vi "BLE v2.0-scalable.vi"(7 "Est Thresh Val":dbl, 8 "Threshold Value Analysis":bool, 9 "Model Name":string="model_name", 10 "Ex_Mod_IDs":string[](array[string]), 11 "Sp_Id_Arr":string[](array[string])) -> (0 "Close 2":bool, 3 "Boolean  Expression":string)   [LabVIEW 2014]
uses:
  <vilib>/Utility/file.llb/Read From Spreadsheet File (string).vi
  <vilib>/Utility/file.llb/Read From Spreadsheet File (DBL).vi
  <vilib>/regexp/Match Regular Expression.xnode
panel:
  out "Input File":path=path "/Volumes/Macintosh HD/Users/hasan/My_MAC_Data/3_Dissemination/DATE 2017/Experimentation/Experimental Results/6Gx78/x78_SSADataLog.xls"
  out "Estimation Time (s)":dbl
  out "Compare":i32[](array[numeric])
  out "element":bool
  out "Output Array":bool[](array[boolean])
  out "Final_BE":string
  out "Int_BE":string
  out "Array 2":bool[][](array[boolean])
  out "Dig_In":bool[](array[boolean])
  out "TV":dbl
  out "Array":u32[](array[numeric])
  out "output variable":i32[](array[numeric])
  out "SD":i32
  out "OP_Var":i32[](array[numeric])
  out "HIGH":i32[](array[numeric])
  out "icv":i32
  out "Case_O":i32[][](array[numeric])
  out "Case_I":i32[](array[numeric])
  out "nc":i32
  out "Input Status":bool
  out "% fitness":string
  out "Simulation Data":string[][](table)
  in  "Close":bool
  out "Row header":string[](array[string])
  out "N":i32
  out "Thresh Val":dbl[](array[numeric])
  out "All Data":string[][](array[string])
  out "Analog Data":dbl[][](array[numeric])
  out "All Data":dbl[][](array[numeric])
  out "Index":i32[](array[numeric])
  out "C1_Ar":dbl[](array[numeric])
  out "C2_Ar":dbl[](array[numeric])
  out "C3_Ar":dbl[](array[numeric])
  out "C4_Ar":dbl[](array[numeric])
  out "Cs4_1s":i32
  out "Cs3_1s":i32
  out "Cs2_1s":i32
  out "Cs1_1s":i32
  out "var_4":i8
  out "var_3":i8
  out "var_2":i8
  out "var_1":i8
  out "case4":i32
  out "case3":i32
  out "case2":i32
  out "case1":i32
  out "C4":dbl
  out "C3":dbl
  out "C2":dbl
  out "C1":dbl
  out "Digital Data":bool[][](array[boolean])
  # "Logic Expression"
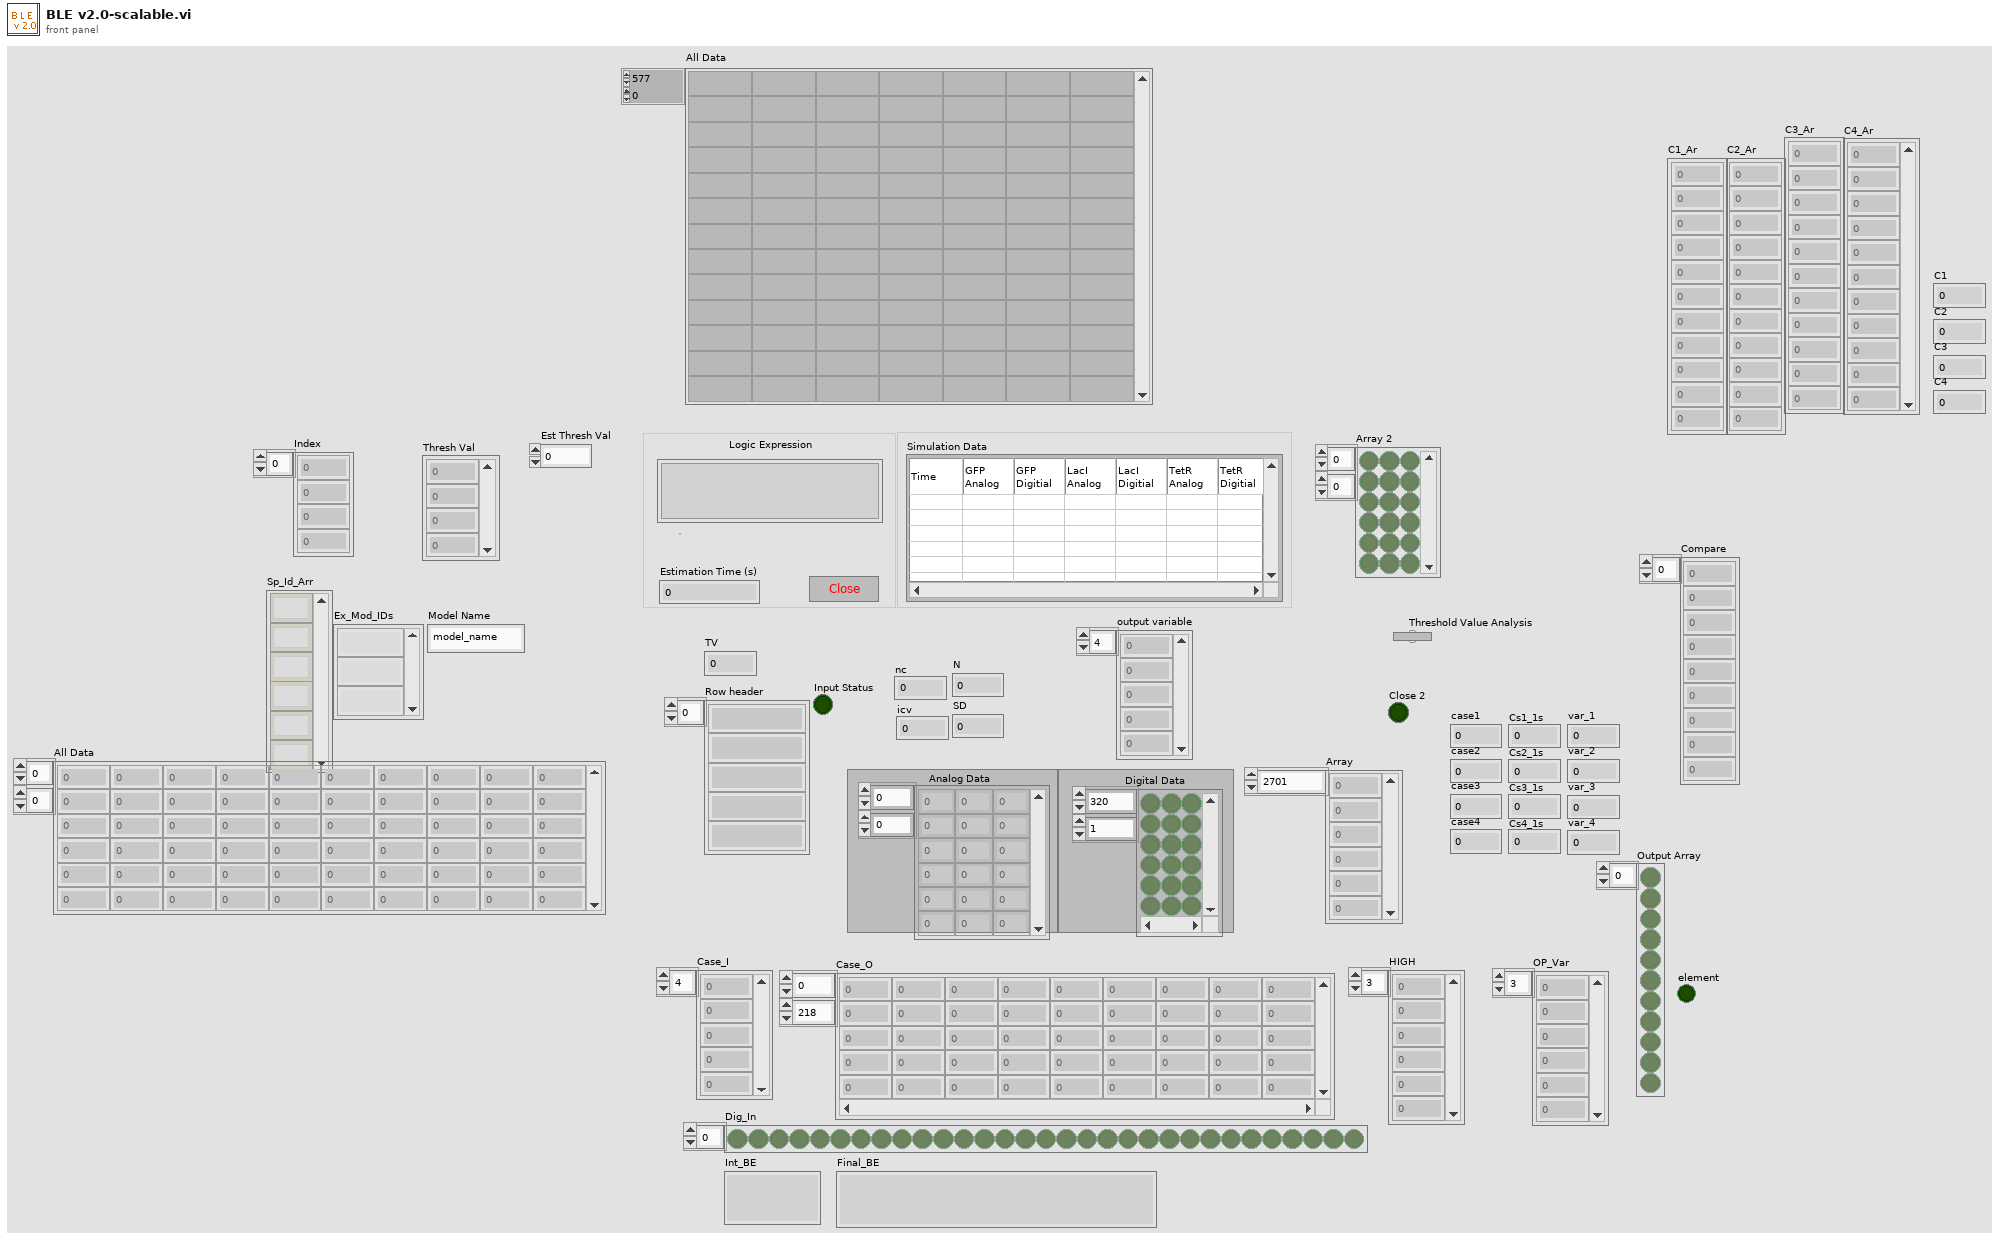
[diagram p1: front panel]
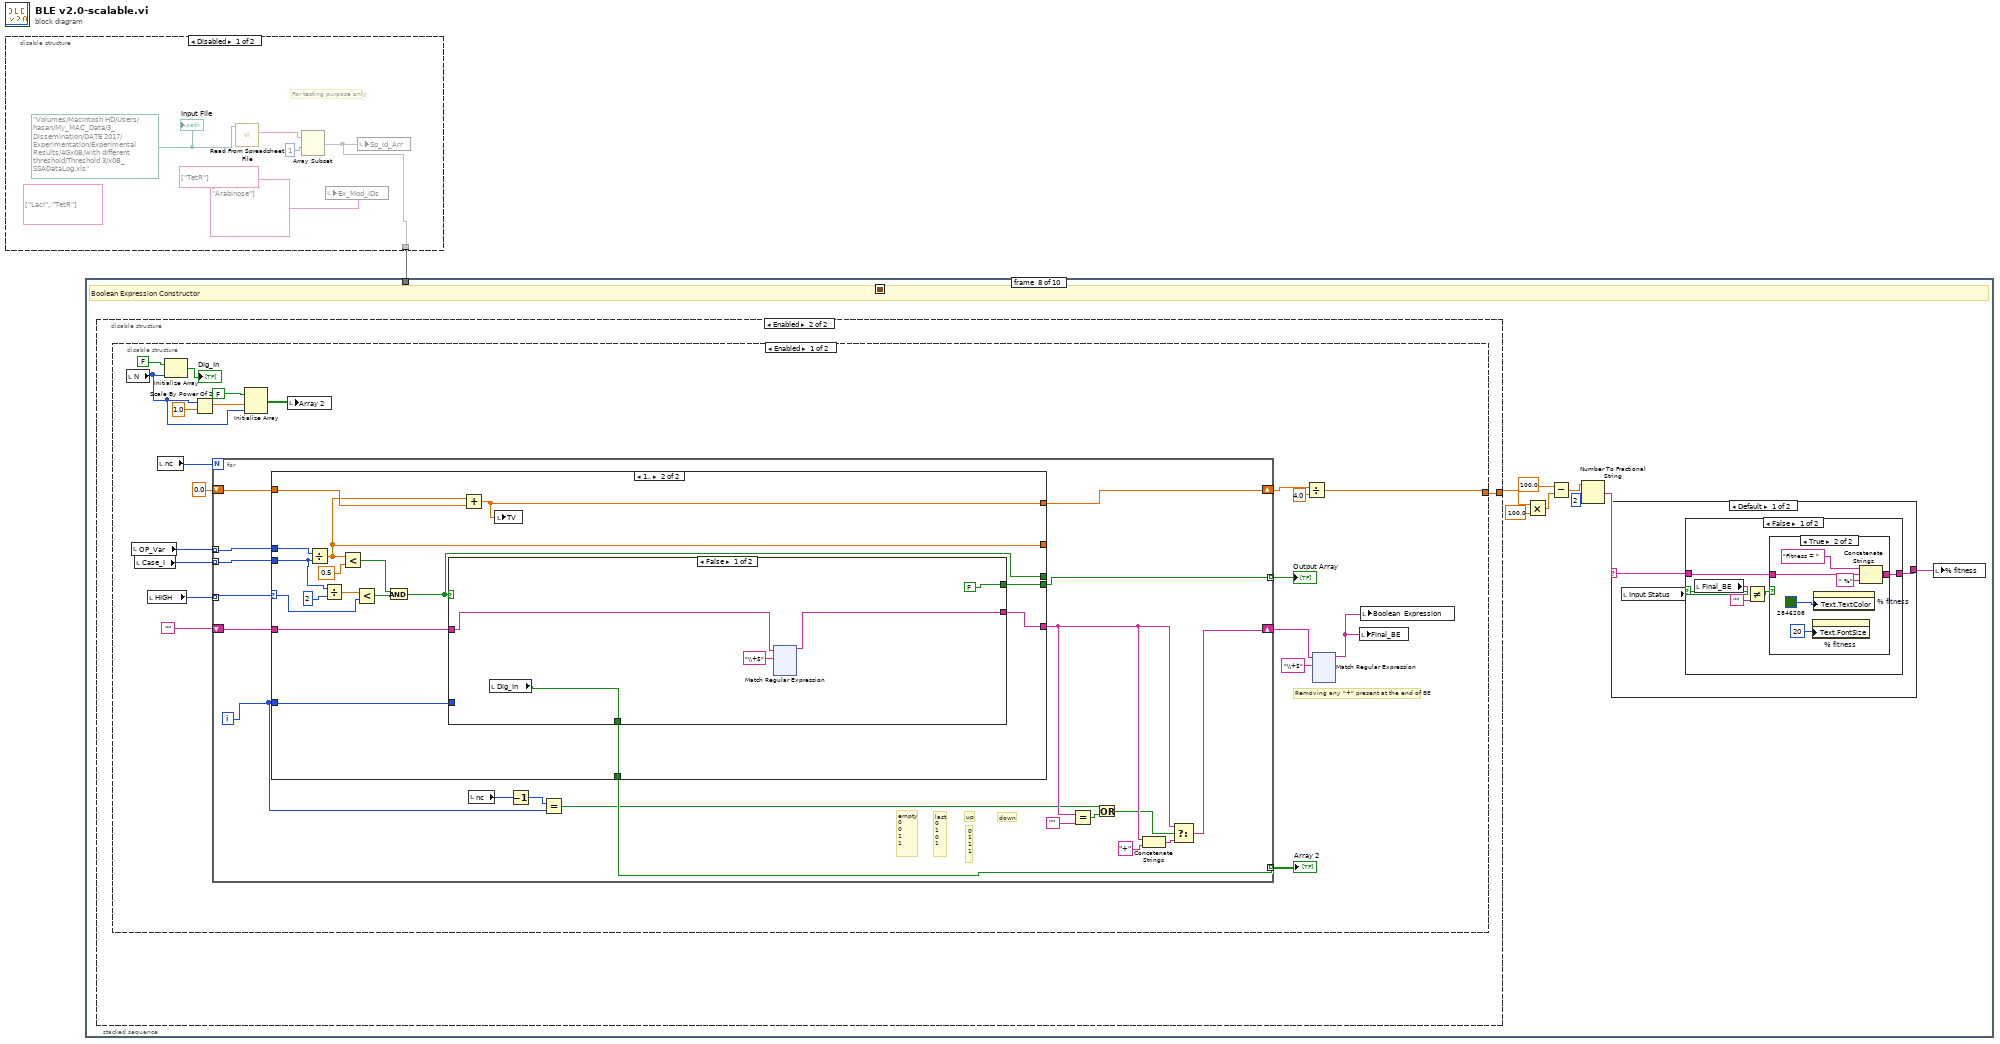
[diagram p0: block diagram]
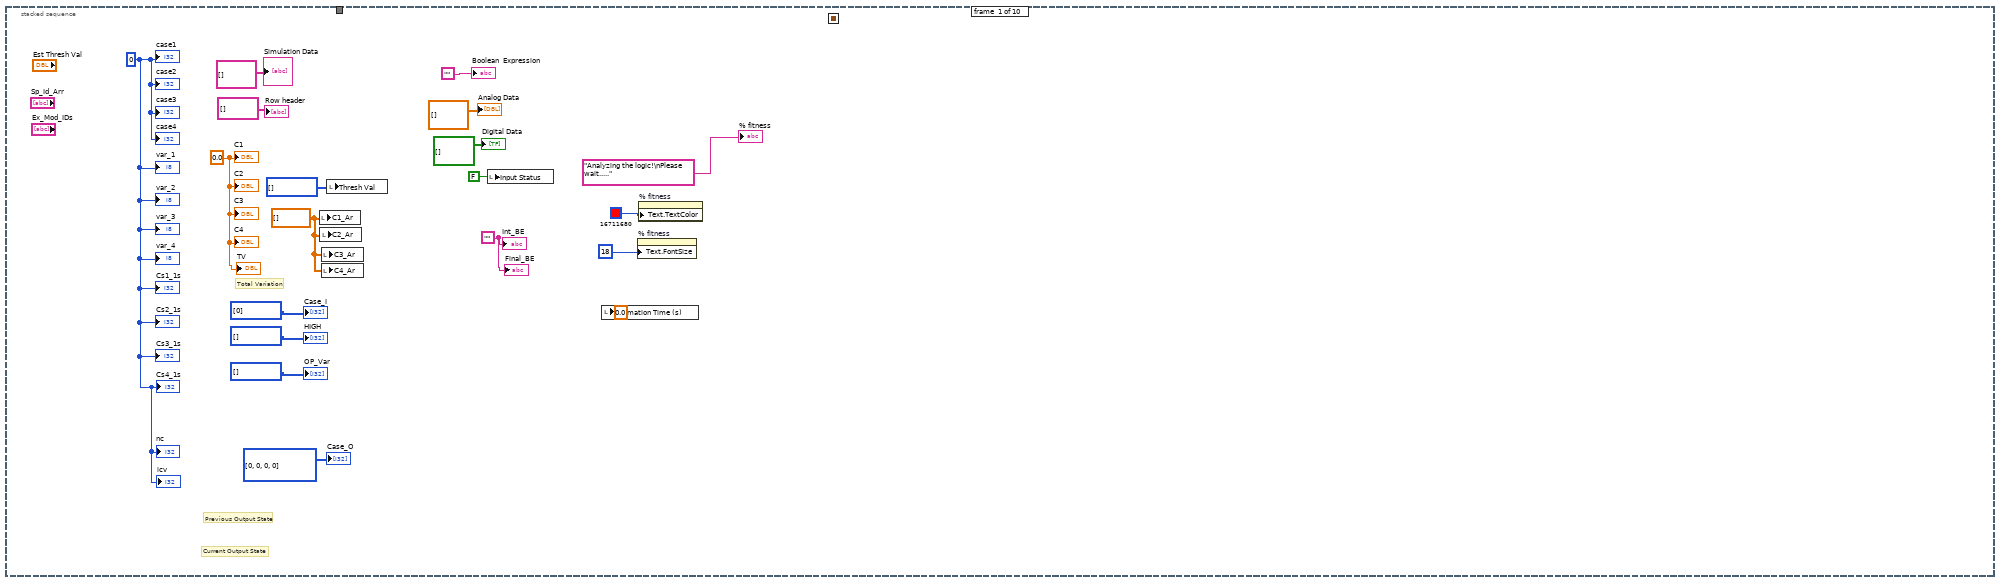
[diagram p3: hidden frame]
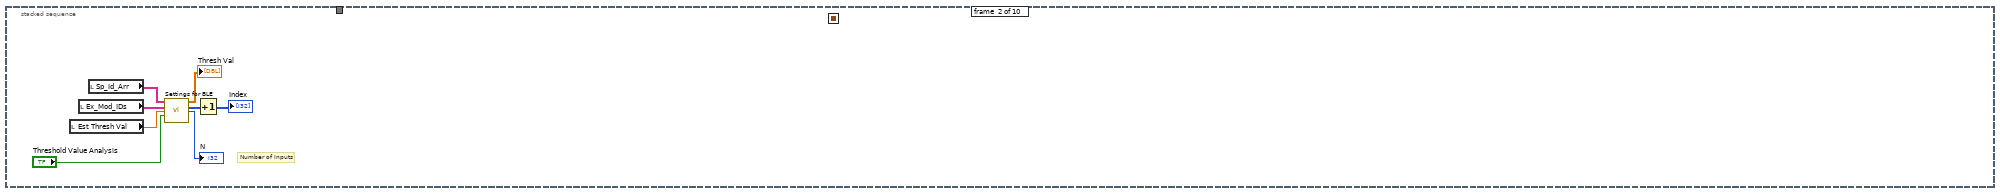
[diagram p4: hidden frame]
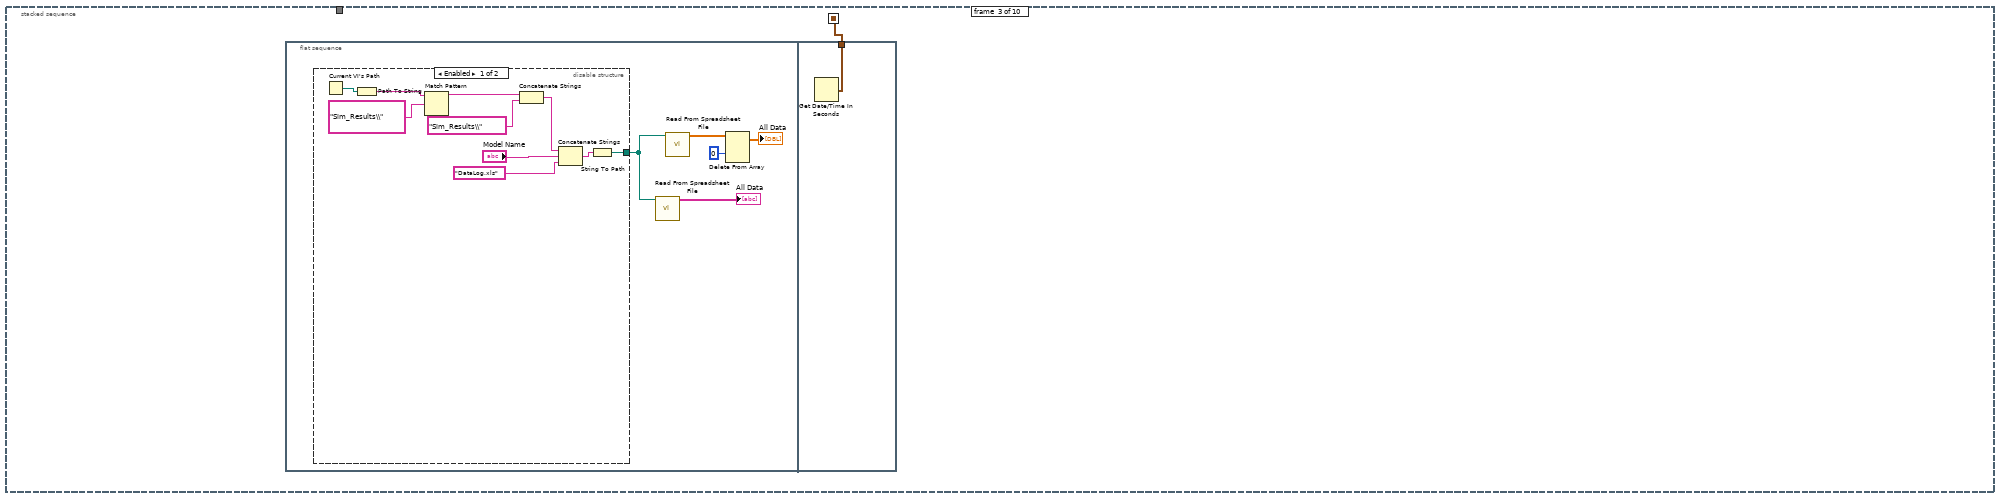
[diagram p5: hidden frame]
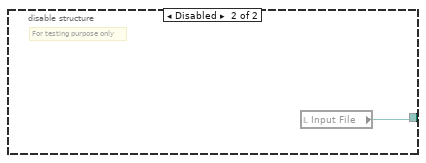
[diagram p6: hidden frame]
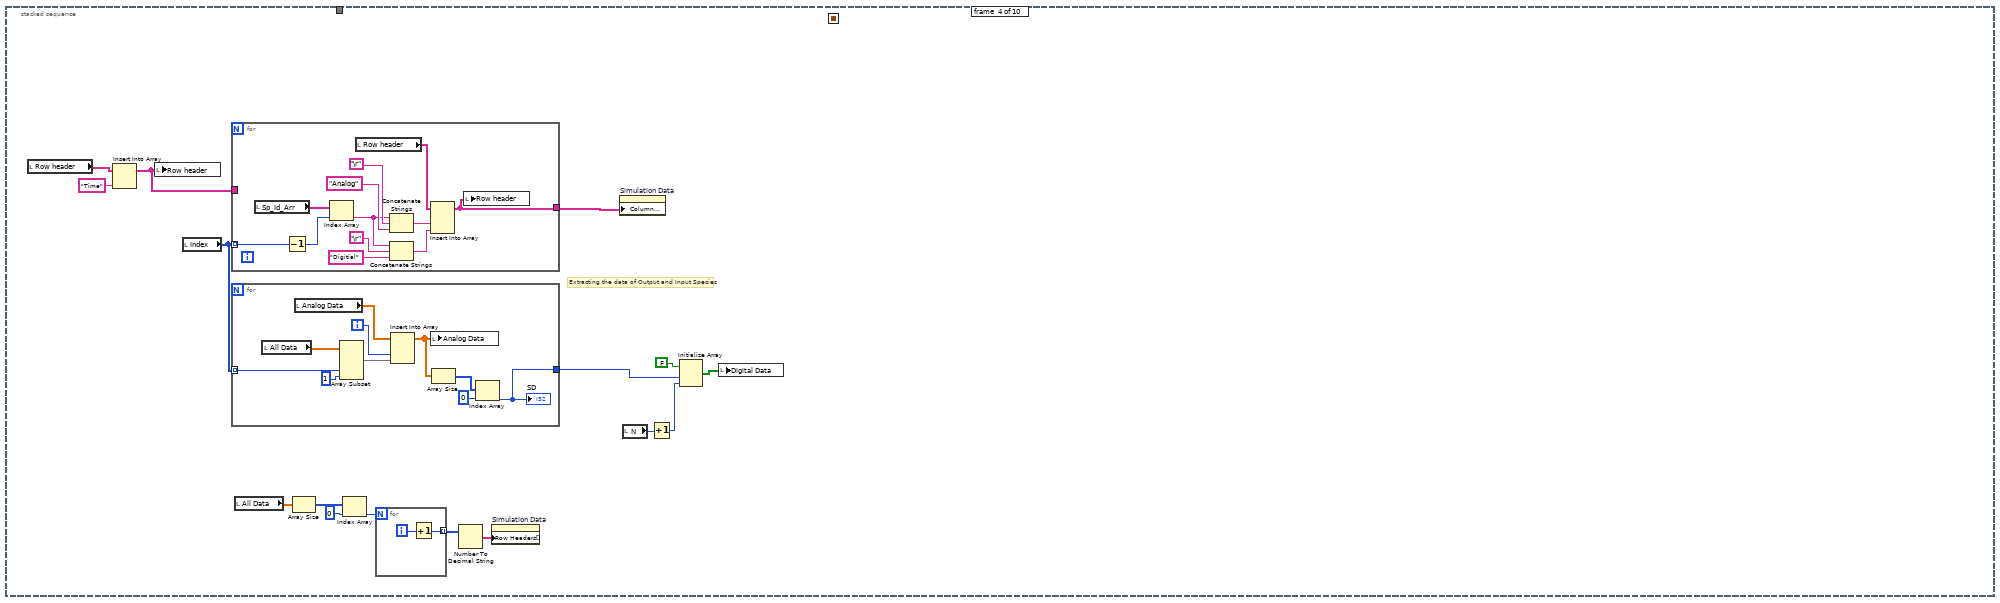
[diagram p7: hidden frame]
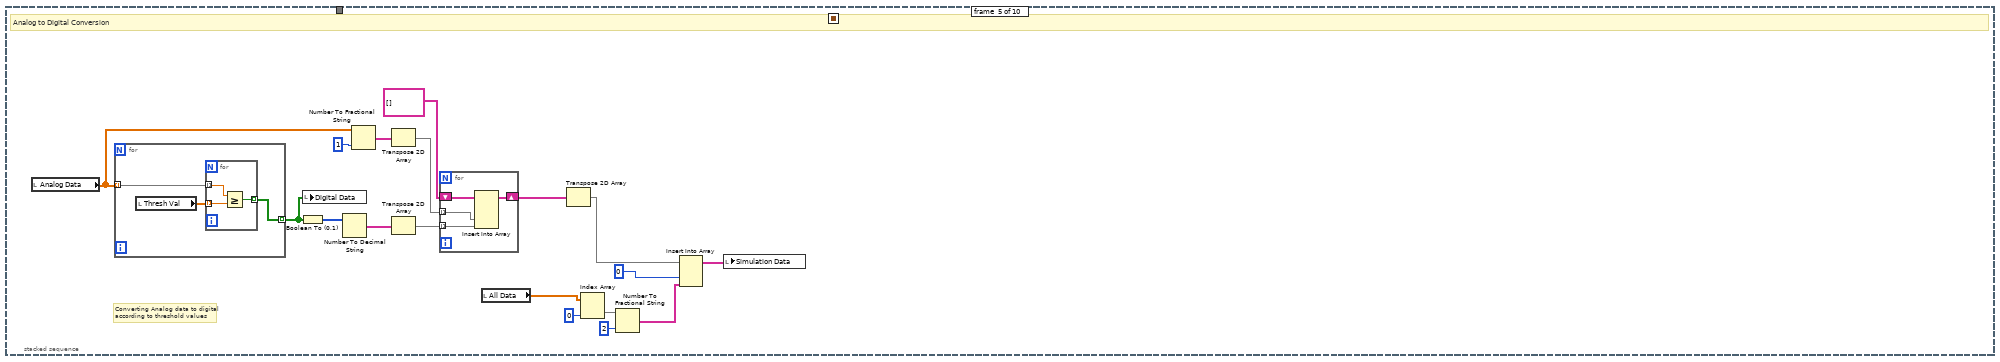
[diagram p8: hidden frame]
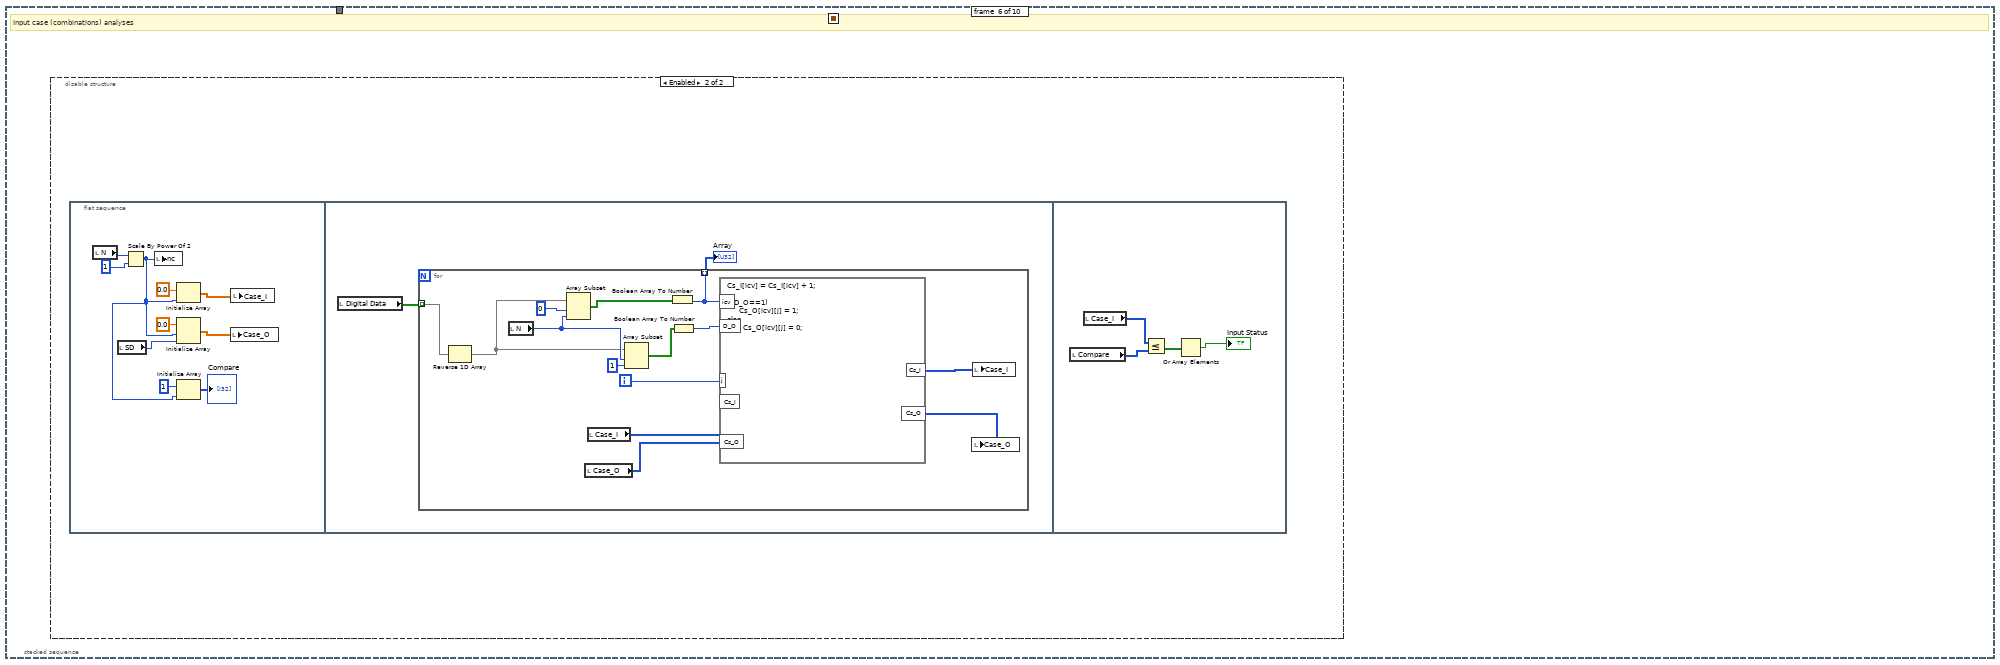
[diagram p9: hidden frame]
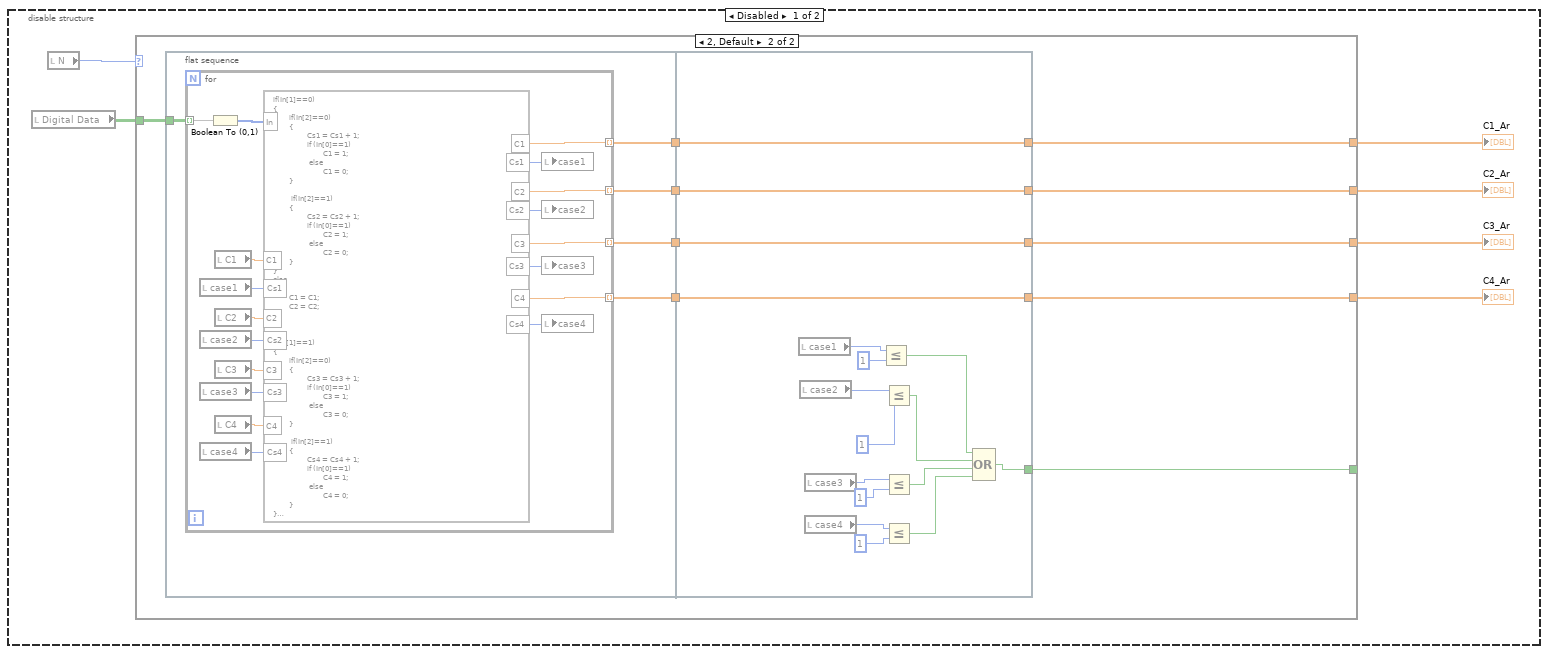
[diagram p10: hidden frame]
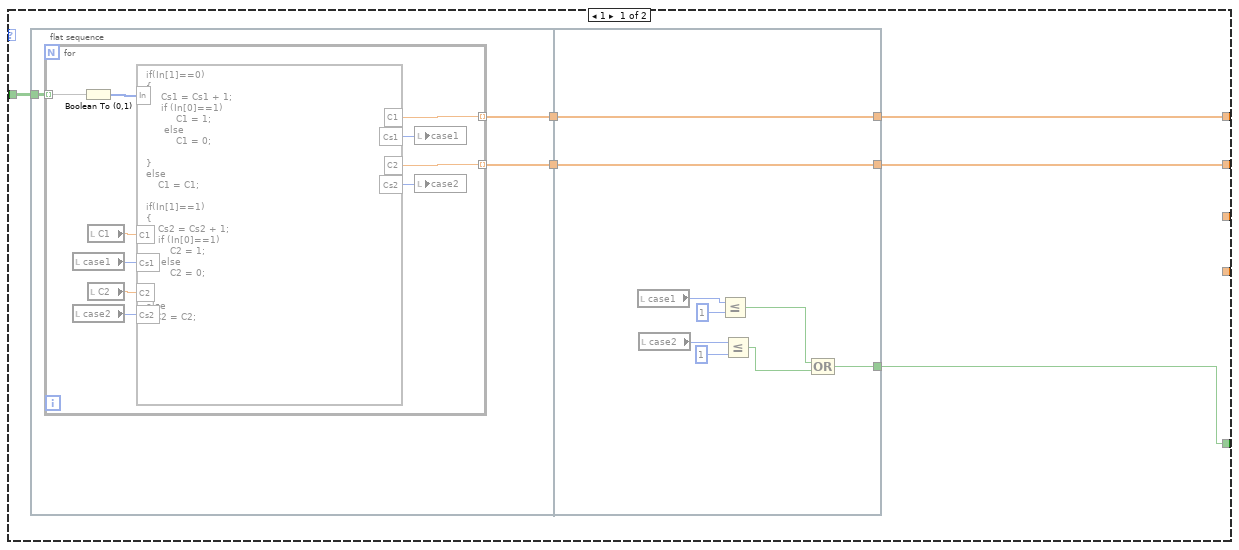
[diagram p11: hidden frame]
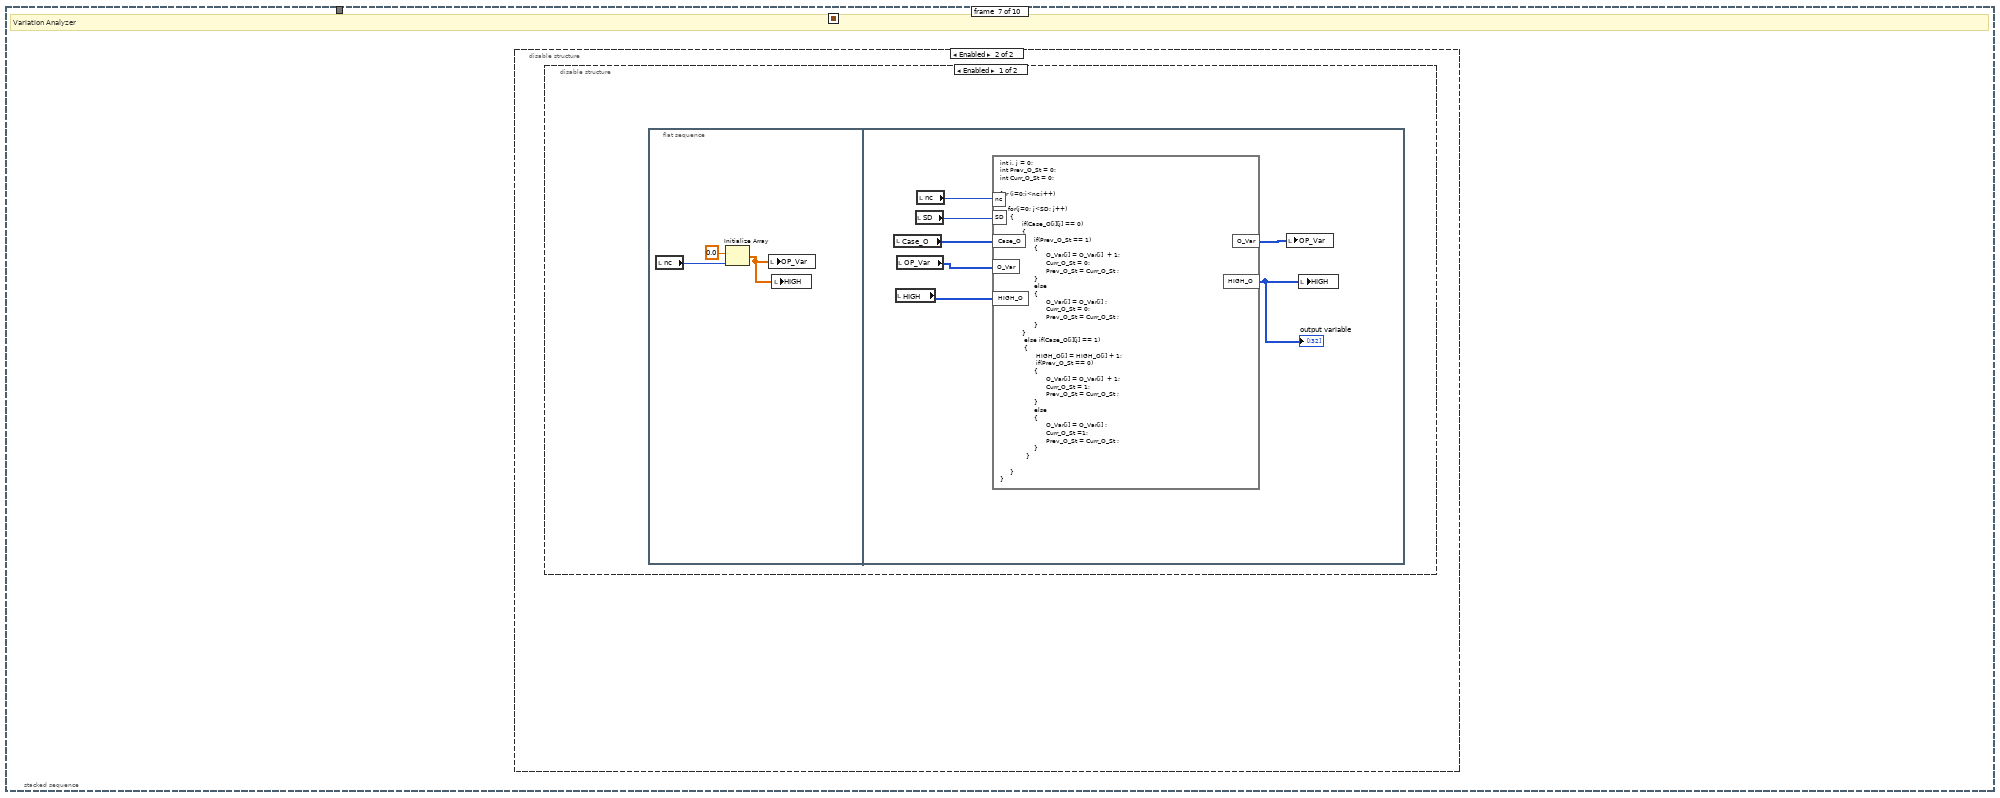
[diagram p12: hidden frame]
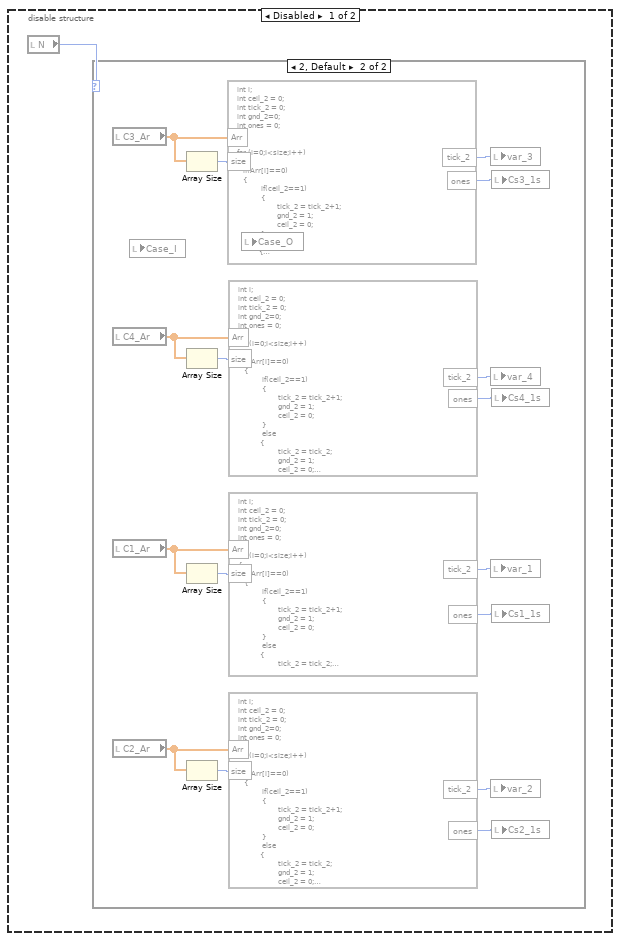
[diagram p13: hidden frame]
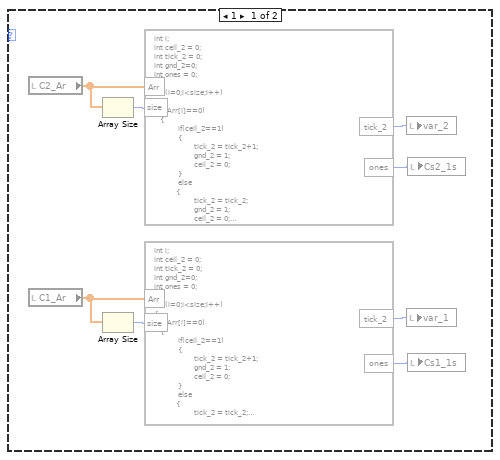
[diagram p14: hidden frame]
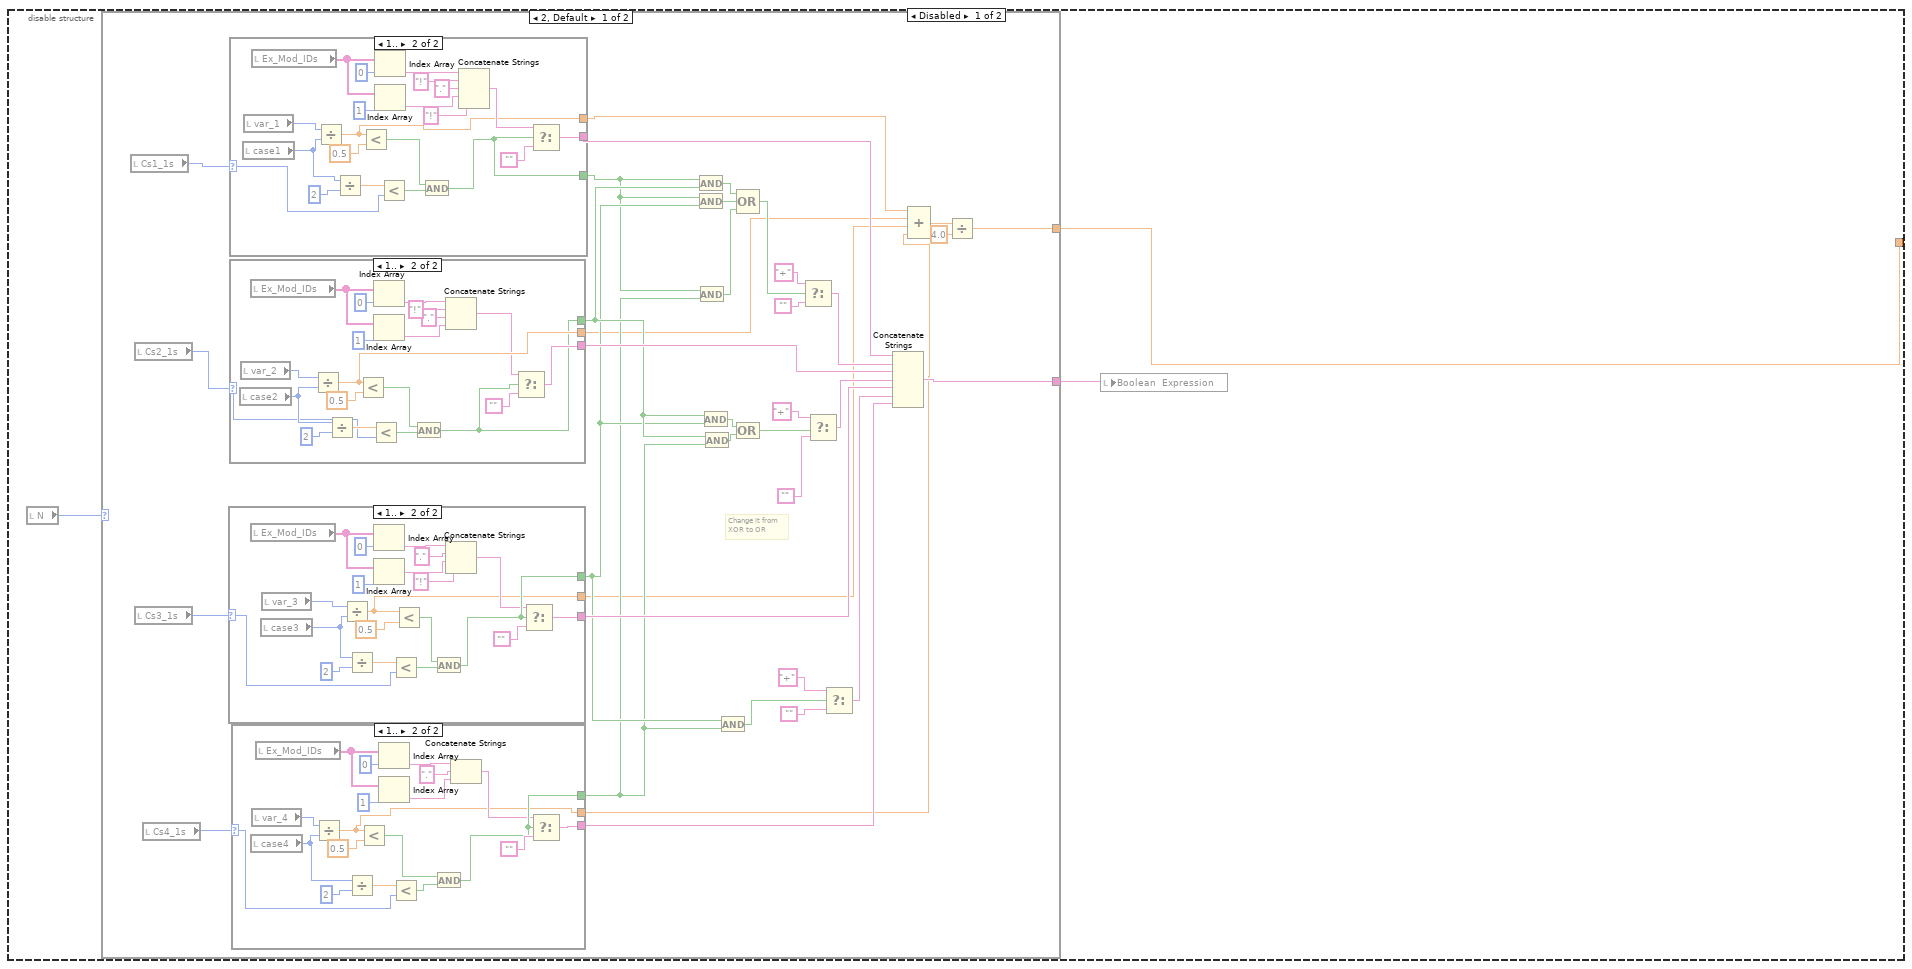
[diagram p16: hidden frame]
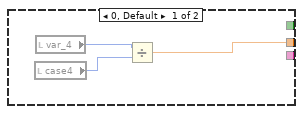
[diagram p17: hidden frame]
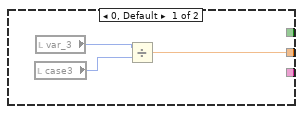
[diagram p18: hidden frame]
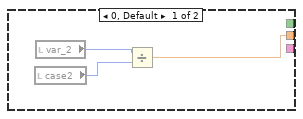
[diagram p19: hidden frame]
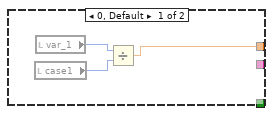
[diagram p20: hidden frame]
diagram:
  n1 = disable-structure shown="Disabled" {
    disable-tunnel: [w3 _] -> w1
    frame Disabled {
      (unwired) string[] ["LacI", "TetR"] ("Ex_Mod_IDs")
      (unwired) string[] ["TetR"] ("Ex_Mod_IDs")
      w6 = path "/Volumes/Macintosh HD/Users/hasan/My_MAC_Data/3_Dissemination/DATE 2017/Experimentation/Experimental Results/4Gx0B/with different threshold/Threshold 3/x0B_SSADataLog.xls"
      # "For testing purpose only"
      n2 = call-poly <vilib>:"Read From Spreadsheet File.vi"("file path (dialog if empty)"=w6) -> ("first row"=w5:string[])  [unwired: 6 in, 4 out]
      n3 = Array Subset(array=w5, index=1) -> (w3:string[])  [unwired: 1 in]
      n4 = local write "Ex_Mod_IDs"(string[] ["IPTG", "aTc", "Arabinose"] ("Ex_Mod_IDs")) -> ()
      n5 = local write "Sp_Id_Arr"(w3) -> ()
      "Input File" <- w6
    }
    frame Enabled {
    }
  }
  n6 = stacked-sequence {
    seq-local: [_ _ w34 _ _ _ _ _ _ _] -> [_ _ _ _ _ _ _ _ _ w1069]
    tunnel: w1 -> [_ _ _ _ _ _ _ _ _ _]
    frame #0 {
      w11 = ""
      w12 = 0.0 ("C1")
      w13 = 0 ("case1")
      w22 = dbl[] [] ("C1_Ar")
      # "Total Variation"
      # "Current Output State"
      # "Previous Output State"
      n7 = local write "C1_Ar"(w22) -> ()
      n8 = local write "C2_Ar"(w22) -> ()
      n9 = local write "C3_Ar"(w22) -> ()
      n10 = local write "C4_Ar"(w22) -> ()
      n11 = local write "Thresh Val"(i32[] [] ("Array")) -> ()
      n12 = local write "Input Status"(FALSE ("Input Status")) -> ()
      n13 = local write "Estimation Time (s)"(0.0 ("x-y")) -> ()
      n14 = property on="% fitness" class="Str"("Text.FontSize"=u32 18 ("Text.Font:Size")) -> ()  [unwired: 2 in, 2 out]
      n15 = property on="% fitness" class="Str"("Text.TextColor"=u32 16711680) -> ()  [unwired: 2 in, 2 out]
      "C1" <- w12
      "C2" <- w12
      "C3" <- w12
      "C4" <- w12
      "case1" <- w13
      "case2" <- w13
      "case3" <- w13
      "case4" <- w13
      "var_1" <- w13
      "var_2" <- w13
      "var_3" <- w13
      "var_4" <- w13
      "Cs1_1s" <- w13
      "Cs2_1s" <- w13
      "Cs3_1s" <- w13
      "Cs4_1s" <- w13
      "Simulation Data" <- string[][] [] ("Table Control")
      "Row header" <- string[] [] ("Row header 2")
      "Digital Data" <- bool[][] [] ("Dig. Data to Process")
      "Boolean  Expression" <- ""
      "Analog Data" <- dbl[][] [] ("Data to process")
      "% fitness" <- "Analyzing the logic!\nPlease wait....." ("% fitness")
      "nc" <- w13
      "Case_I" <- i32[] [0] ("Array")
      "Case_O" <- i32[][] [[0, 0], [0, 0]] ("Array")
      "icv" <- w13
      "HIGH" <- i32[] [] ("Array")
      "OP_Var" <- i32[] [] ("Array")
      "TV" <- w12
      "Int_BE" <- w11
      "Final_BE" <- w11
    }
    frame #1 {
      # "Number of Inputs"
      n16 = local read "Est Thresh Val"() -> (w27:dbl)
      n17 = local read "Ex_Mod_IDs"() -> (w32:string[])
      n18 = local read "Sp_Id_Arr"() -> (w33:string[])
      n19 = call "Settings for BLE.vi"("Sp_Id_Arr"=w33, "Ex_Mod_IDs"=w32, "Est Thresh Val"=w27, "Threshold Value Analysis"="Threshold Value Analysis") -> ("Thresh Val"=→"Thresh Val":dbl[], "Index"=w31:i32[], "No of I/ps"=→"N":i32)  [unwired: 9 in]
      n20 = Increment(x=w31) -> (x+1=→"Index":i32[])
    }
    frame #2 {
      n21 = flat-sequence {
        tunnel: [w51] -> w34
        frame #0 {
          n22 = disable-structure shown="Enabled" {
            disable-tunnel: [w49 w50] -> w39
            frame Enabled {
              n23 = Current VI's Path() -> (path=w46:path)
              n24 = Path To String(path=w46) -> (string=w45:string)
              n25 = Match Pattern(string=w45, regular expression="Sim_Results\\" ("string")) -> (before substring=w43:string)  [unwired: 1 in, 3 out]
              n26 = Concatenate Strings(w43, "Sim_Results\\" ("string")) -> (w47:string)
              n27 = Concatenate Strings(w47, "Model Name", "DataLog.xls" ("name or relative path")) -> (w48:string)
              n28 = String To Path(string=w48) -> (path=w49:path)
            }
            frame Disabled {
              # "For testing purpose only"
              n29 = local read "Input File"() -> (w50:path)
            }
          }
          n30 = call-poly <vilib>:"Read From Spreadsheet File.vi"("file path (dialog if empty)"=w39) -> ("all rows"=→"All Data":string[][])  [unwired: 6 in, 4 out]
          n31 = call-poly <vilib>:"Read From Spreadsheet File.vi"("file path (dialog if empty)"=w39) -> ("all rows"=w38:dbl[][])  [unwired: 6 in, 4 out]
          n32 = Delete From Array(array=w38, index (row)=0) -> (array with subset deleted=→"All Data":dbl[][])  [unwired: 2 in, 1 out]
        }
        frame #1 {
          n33 = Get Date/Time In Seconds() -> (seconds since 1Jan1904=w51:timestamp)
        }
      }
    }
    frame #3 {
      # "Extracting the data of Output and Input Species"
      n34 = local read "Row header"() -> (w58:string[])
      n35 = Insert Into Array(array=w58, new element="Time" ("new element/subarray")) -> (w59:string[])  [unwired: 1 in]
      n36 = local write "Row header"(w59) -> ()
      n37 = local read "Index"() -> (w67:i32[])
      n38 = for {
        tunnel: w67 -> [w80] mode=indexing
        tunnel: [w71] -> w66
        tunnel: w59 -> [_]
        n39 = local read "Sp_Id_Arr"() -> (w81:string[])
        n40 = Decrement(x=w80) -> (x-1=w79:i32)
        n41 = Index Array(array=w81, index=w79) -> (element=w73:string)
        n42 = local read "Row header"() -> (w70:string[])
        n43 = Concatenate Strings(w73, "\r", "Analog" ("string")) -> (w76:string)
        n44 = Concatenate Strings(w73, "\r", "Digitial" ("string")) -> (w72:string)
        n45 = Insert Into Array(array=w70, new element #1=w76, new element #2=w72) -> (w71:string[])  [unwired: 1 in]
        n46 = local write "Row header"(w71) -> ()
      }
      n47 = for {
        tunnel: w67 -> [w90] mode=indexing
        tunnel: [w82] -> w52
        i -> [w87]
        n48 = local read "All Data"() -> (w91:dbl[][])
        n49 = local read "Analog Data"() -> (w86:dbl[][])
        n50 = Array Subset(array=w91, index (col)=w90, length (col)=1 ("length")) -> (w88:dbl[][])  [unwired: 2 in]
        n51 = Insert Into Array(array=w86, index (col)=w87, new element=w88) -> (w83:dbl[][])  [unwired: 1 in]
        n52 = local write "Analog Data"(w83) -> ()
        n53 = Array Size(array=w83) -> (size(s)=w84:i32[])
        n54 = Index Array(array=w84, index=0) -> (element=w82:i32)
        "SD" <- w82
      }
      n55 = local read "All Data"() -> (w65:dbl[][])
      n56 = Array Size(array=w65) -> (size(s)=w64:i32[])
      n57 = Index Array(array=w64, index=0) -> (element=w62:i32)
      n58 = for {
        N: w62 -> [_]
        tunnel: [w68] -> w61 mode=indexing
        i -> [w69]
        n59 = Increment(x=w69) -> (x+1=w68:i32)
      }
      n60 = Number To Decimal String(number=w61) -> (decimal integer string=w60:string[])  [unwired: 1 in]
      n61 = property on="Simulation Data" class="Tbl (strict)"("Row Headers[]"=w60) -> ()  [unwired: 2 in, 2 out]
      n62 = property on="Simulation Data" class="Tbl (strict)"("Column Headers[]"=w66) -> ()  [unwired: 2 in, 2 out]
      n63 = local read "N"() -> (w55:i32)
      n64 = Increment(x=w55) -> (x+1=w54:i32)
      n65 = Initialize Array(FALSE, w52, w54) -> (w56:bool[][])
      n66 = local write "Digital Data"(w56) -> ()
    }
    frame #4 {
      # "Converting Analog data to digital\naccording to threshold values"
      # "Analog to Digital Conversion"
      n67 = local read "Analog Data"() -> (w106:dbl[][])
      n68 = for {
        tunnel: w106 -> [w115] mode=indexing
        tunnel: [w114] -> w92 mode=indexing
        n69 = local read "Thresh Val"() -> (w116:dbl[])
        n70 = for {
          tunnel: w115 -> [w118] mode=indexing
          tunnel: w116 -> [w119] mode=indexing
          tunnel: [w117] -> w114 mode=indexing
          n71 = Greater Or Equal?(x=w118, y=w119) -> (x >= y?=w117:bool)
        }
      }
      n72 = Boolean To (0,1)(Boolean=w92) -> (0, 1=w108:i16[][])
      n73 = local write "Digital Data"(w92) -> ()
      n74 = Number To Decimal String(number=w108) -> (decimal integer string=w103:string[][])  [unwired: 1 in]
      n75 = Number To Fractional String(number=w106, precision (6)=i16 1) -> (F-format string=w105:string[][])  [unwired: 2 in]
      n76 = Transpose 2D Array(2D array=w105) -> (transposed array=w104:string[][])
      n77 = Transpose 2D Array(2D array=w103) -> (transposed array=w102:string[][])
      n78 = for {
        shift-right: [w113] -> w101
        shift-left: string[][] [] -> [w112]
        tunnel: w102 -> [w111] mode=indexing
        tunnel: w104 -> [w110] mode=indexing
        n79 = Insert Into Array(array=w112, new element #1=w110, new element #2=w111) -> (w113:string[][])  [unwired: 2 in]
      }
      n80 = local read "All Data"() -> (w99:dbl[][])
      n81 = Transpose 2D Array(2D array=w101) -> (transposed array=w100:string[][])
      n82 = Index Array(array=w99, index (col)=0 ("disabled index (col)")) -> (element=w97:dbl[])  [unwired: 1 in]
      n83 = Number To Fractional String(number=w97, precision (6)=i16 2) -> (F-format string=w95:string[])  [unwired: 2 in]
      n84 = Insert Into Array(array=w100, index (col)=0 ("disabled index (col)"), new element=w95) -> (w93:string[][])  [unwired: 1 in]
      n85 = local write "Simulation Data"(w93) -> ()
    }
    frame #5 {
      # "Input case (combinations) analyses"
      n86 = disable-structure shown="Enabled" {
        frame Disabled {
          n87 = local read "Digital Data"() -> (w126:bool[][])
          n88 = local read "N"() -> (w121:i32)
          n89 = case shown="2, Default" w121 {
            tunnel: w126 -> [w132 w164]
            tunnel: [w130 w163] -> w125
            tunnel: [w131 w162] -> w124
            tunnel: [_ w161] -> w123
            tunnel: [_ w160] -> w122
            tunnel: [w127 w155] -> w120
            frame 1 {
              n90 = flat-sequence {
                tunnel: w132 -> [w135]
                tunnel: [w134] -> w129
                tunnel: [w133] -> w128
                tunnel: [w153] -> w130
                tunnel: [w154] -> w131
                tunnel: w129 -> [w154]
                tunnel: w128 -> [w153]
                tunnel: [w146] -> w127
                frame #0 {
                  n91 = for {
                    tunnel: [w138] -> w133 mode=indexing
                    tunnel: [w137] -> w134 mode=indexing
                    tunnel: w135 -> [w136] mode=indexing
                    n92 = local read "case1"() -> (w143:i32)
                    n93 = local read "case2"() -> (w142:i32)
                    n94 = Boolean To (0,1)(Boolean=w136) -> (0, 1=w145:i16[])
                    n95 = local read "C1"() -> (w141:dbl)
                    n96 = local read "C2"() -> (w144:dbl)
                    n97 = formula code="if(In[1]==0)\n{\n     Cs1 = Cs1 + 1;\n     if (In[0]==1)\n          C1 = 1;\n      else\n          C1 = 0;\n\n}\nelse\n    C1 = C1;\n\nif(In[1]==1)\n{\n    Cs2 = Cs2 + 1;\n    if (In[0]==1)\n        C2 = 1;\n     else\n        C2 = 0;\n\n}\nelse\n   C2 = C2;"("In"=w145, "C1"=w141, "C2"=w144, "Cs1"=w143, "Cs2"=w142) -> ("C1"=w138:dbl, "C2"=w137:dbl, "Cs1"=w139:i32, "Cs2"=w140:i32)
                    n98 = local write "case1"(w139) -> ()
                    n99 = local write "case2"(w140) -> ()
                  }
                }
                frame #1 {
                  n100 = local read "case1"() -> (w152:i32)
                  n101 = local read "case2"() -> (w148:i32)
                  n102 = Less Or Equal?(x=w152, y=1) -> (x <= y?=w150:bool)
                  n103 = Less Or Equal?(x=w148, y=1) -> (x <= y?=w151:bool)
                  n104 = Compound Arithmetic op=OR(w150, w151) -> (w146:bool)
                }
              }
            }
            frame 2, Default {
              n105 = flat-sequence {
                tunnel: w164 -> [w169]
                tunnel: [w168] -> w159
                tunnel: [w167] -> w158
                tunnel: [w166] -> w157
                tunnel: [w165] -> w156
                tunnel: [w201] -> w160
                tunnel: [w202] -> w161
                tunnel: [w203] -> w162
                tunnel: [w204] -> w163
                tunnel: w159 -> [w204]
                tunnel: w158 -> [w203]
                tunnel: w157 -> [w202]
                tunnel: w156 -> [w201]
                tunnel: [w188] -> w155
                frame #0 {
                  n106 = for {
                    tunnel: w169 -> [w187] mode=indexing
                    tunnel: [w173] -> w168 mode=indexing
                    tunnel: [w172] -> w167 mode=indexing
                    tunnel: [w171] -> w166 mode=indexing
                    tunnel: [w170] -> w165 mode=indexing
                    n107 = local read "case1"() -> (w182:i32)
                    n108 = local read "case2"() -> (w179:i32)
                    n109 = local read "case3"() -> (w181:i32)
                    n110 = local read "case4"() -> (w180:i32)
                    n111 = Boolean To (0,1)(Boolean=w187) -> (0, 1=w186:i16[])
                    n112 = local read "C1"() -> (w178:dbl)
                    n113 = local read "C2"() -> (w185:dbl)
                    n114 = local read "C3"() -> (w184:dbl)
                    n115 = local read "C4"() -> (w183:dbl)
                    n116 = formula code="if(In[1]==0)\n{\n        if(In[2]==0)\n        {\n                 Cs1 = Cs1 + 1;\n                 if (In[0]==1)\n                         C1 = 1;\n                  else\n                         C1 = 0;\n        }\n\n         if(In[2]==1)\n        {\n                 Cs2 = Cs2 + 1;\n                 if (In[0]==1)\n                         C2 = 1;\n                  else\n                         C2 = 0;\n        }  \n}\nelse\n{\n        C1 = C1;\n        C2 = C2;\n}\n\n\nif(In[1]==1)\n{\n        if(In[2]==0)\n        {\n                 Cs3 = Cs3 + 1;\n                 if (In[0]==1)\n                         C3 = 1;\n                  else\n                         C3 = 0;\n        }\n\n         if(In[2]==1)\n        {\n                 Cs4 = Cs4 + 1;\n                 if (In[0]==1)\n                         C4 = 1;\n                  else\n                         C4 = 0;\n        }  \n}\nelse\n{\n        C3 = C3;\n        C4 = C4;\n}"("In"=w186, "C1"=w178, "C2"=w185, "C3"=w184, "C4"=w183, "Cs1"=w182, "Cs2"=w179, "Cs3"=w181, "Cs4"=w180) -> ("C1"=w173:dbl, "C2"=w172:dbl, "C3"=w171:dbl, "C4"=w170:dbl, "Cs1"=w174:i32, "Cs2"=w175:i32, "Cs3"=w176:i32, "Cs4"=w177:i32)
                    n117 = local write "case1"(w174) -> ()
                    n118 = local write "case2"(w175) -> ()
                    n119 = local write "case3"(w176) -> ()
                    n120 = local write "case4"(w177) -> ()
                  }
                }
                frame #1 {
                  n121 = local read "case1"() -> (w200:i32)
                  n122 = local read "case2"() -> (w190:i32)
                  n123 = local read "case3"() -> (w193:i32)
                  n124 = local read "case4"() -> (w194:i32)
                  n125 = Less Or Equal?(x=w200, y=1) -> (x <= y?=w196:bool)
                  n126 = Less Or Equal?(x=w190, y=1) -> (x <= y?=w197:bool)
                  n127 = Less Or Equal?(x=w193, y=1) -> (x <= y?=w198:bool)
                  n128 = Less Or Equal?(x=w194, y=1) -> (x <= y?=w199:bool)
                  n129 = Compound Arithmetic op=OR(w196, w197, w198, w199) -> (w188:bool)
                }
              }
            }
          }
          "C1_Ar" <- w125
          "C2_Ar" <- w124
          "C3_Ar" <- w123
          "C4_Ar" <- w122
        }
        frame Enabled {
          n130 = flat-sequence {
            frame #0 {
              n131 = local read "N"() -> (w208:i32)
              n132 = local read "SD"() -> (w214:i32)
              n133 = Scale By Power Of 2(n=w208, x=1 ("N")) -> (x*2^n=w205:i32)
              n134 = local write "nc"(w205) -> ()
              n135 = Initialize Array(0.0 ("element"), w205) -> (w211:dbl[])
              n136 = Initialize Array(0.0 ("element"), w205, w214) -> (w213:dbl[][])
              n137 = Initialize Array(1 ("element"), w205) -> (→"Compare":i32[])
              n138 = local write "Case_O"(w213) -> ()
              n139 = local write "Case_I"(w211) -> ()
            }
            frame #1 {
              n140 = local read "Digital Data"() -> (w216:bool[][])
              n141 = for {
                tunnel: w216 -> [w221] mode=indexing
                tunnel: [w222] -> w215 mode=indexing
                i -> [w225]
                n142 = Reverse 1D Array(array=w221) -> (reversed array=w217:bool[])
                n143 = local read "N"() -> (w219:i32)
                n144 = Array Subset(array=w217, index=0, length=w219) -> (w218:bool[])
                n145 = local read "Case_O"() -> (w226:i32[][])
                n146 = local read "Case_I"() -> (w230:i32[])
                n147 = Array Subset(array=w217, index=w219, length=1) -> (w228:bool[])
                n148 = Boolean Array To Number(Boolean array=w218) -> (number=w222:u32)
                n149 = Boolean Array To Number(Boolean array=w228) -> (number=w223:u32)
                n150 = formula code="Cs_I[icv] = Cs_I[icv] + 1; \n\nif(D_O==1)\n      Cs_O[icv][j] = 1;\nelse\n        Cs_O[icv][j] = 0;"("icv"=w222, "j"=w225, "Cs_I"=w230, "Cs_O"=w226, "D_O"=w223) -> ("Cs_I"=w227:i32[], "Cs_O"=w224:i32[][])
                n151 = local write "Case_O"(w224) -> ()
                n152 = local write "Case_I"(w227) -> ()
              }
              "Array" <- w215
            }
            frame #2 {
              n153 = local read "Compare"() -> (w233:i32[])
              n154 = local read "Case_I"() -> (w234:i32[])
              n155 = Less Or Equal?(x=w234, y=w233) -> (x <= y?=w232:bool[])
              n156 = Or Array Elements(Boolean array=w232) -> (logical OR=→"Input Status":bool)
            }
          }
        }
      }
    }
    frame #6 {
      # "Variation Analyzer"
      n157 = disable-structure shown="Enabled" {
        frame Disabled {
          n158 = local read "N"() -> (w235:i32)
          n159 = case shown="2, Default" w235 {
            frame 1 {
              n160 = local read "C2_Ar"() -> (w240:dbl[])
              n161 = local read "C1_Ar"() -> (w241:dbl[])
              n162 = Array Size(array=w240) -> (size(s)=w242:i32)
              n163 = Array Size(array=w241) -> (size(s)=w243:i32)
              n164 = formula code="int i;\nint ceil_2 = 0;\nint tick_2 = 0;\nint gnd_2=0;\nint ones = 0;\n\nfor (i=0;i<size;i++)\n{\n   if(Arr[i]==0)\n   { \n            if(ceil_2==1)\n            {\n                    tick_2 = tick_2+1;\n                    gnd_2 = 1;\n                    ceil_2 = 0;\n            }\n            else \n           {\n                    tick_2 = tick_2;\n                    gnd_2 = 1;\n                    ceil_2 = 0;                 \n           } \n   }\n   \n   else if(Arr[i]==1)\n   {\n            ones = ones +1;\n            if(gnd_2==1)\n            {\n                    tick_2 = tick_2+1;\n                    gnd_2 = 0;\n                    ceil_2 = 1;\n            }\n            else \n           {\n                    tick_2 = tick_2;\n                    gnd_2 = gnd_2;\n                    ceil_2 = 1;                 \n           } \n   }\n   else\n   {\n           tick_2 = tick_2;\n           ceil_2 = ceil_2;\n           gnd_2 = gnd_2;\n   }\n}"("Arr"=w240, "size"=w242) -> ("tick_2"=w237:i32, "ones"=w236:i32)
              n165 = formula code="int i;\nint ceil_2 = 0;\nint tick_2 = 0;\nint gnd_2=0;\nint ones = 0;\n\nfor (i=0;i<size;i++)\n{\n   if(Arr[i]==0)\n   { \n            if(ceil_2==1)\n            {\n                    tick_2 = tick_2+1;\n                    gnd_2 = 1;\n                    ceil_2 = 0;\n            }\n            else \n           {\n                    tick_2 = tick_2;\n                    gnd_2 = 1;\n                    ceil_2 = 0;                 \n           } \n   }\n   \n   else if(Arr[i]==1)\n   {\n            ones = ones +1;\n            if(gnd_2==1)\n            {\n                    tick_2 = tick_2+1;\n                    gnd_2 = 0;\n                    ceil_2 = 1;\n            }\n            else \n           {\n                    tick_2 = tick_2;\n                    gnd_2 = gnd_2;\n                    ceil_2 = 1;                 \n           } \n   }\n   else\n   {\n           tick_2 = tick_2;\n           ceil_2 = ceil_2;\n           gnd_2 = gnd_2;\n   }\n}"("Arr"=w241, "size"=w243) -> ("tick_2"=w239:i32, "ones"=w238:i32)
              n166 = local write "var_2"(w237) -> ()
              n167 = local write "var_1"(w239) -> ()
              n168 = local write "Cs2_1s"(w236) -> ()
              n169 = local write "Cs1_1s"(w238) -> ()
            }
            frame 2, Default {
              n170 = local read "C3_Ar"() -> (w252:dbl[])
              n171 = local read "C4_Ar"() -> (w254:dbl[])
              n172 = local read "C1_Ar"() -> (w255:dbl[])
              n173 = local read "C2_Ar"() -> (w253:dbl[])
              n174 = local read "Case_I"() -> ()  [unwired: 1 in]
              n175 = Array Size(array=w252) -> (size(s)=w258:i32)
              n176 = Array Size(array=w254) -> (size(s)=w256:i32)
              n177 = Array Size(array=w255) -> (size(s)=w259:i32)
              n178 = Array Size(array=w253) -> (size(s)=w257:i32)
              n179 = formula code="int i;\nint ceil_2 = 0;\nint tick_2 = 0;\nint gnd_2=0;\nint ones = 0;\n\n\nfor (i=0;i<size;i++)\n{\n   if(Arr[i]==0)\n   { \n            if(ceil_2==1)\n            {\n                    tick_2 = tick_2+1;\n                    gnd_2 = 1;\n                    ceil_2 = 0;\n            }\n            else \n           {\n                    tick_2 = tick_2;\n                    gnd_2 = 1;\n                    ceil_2 = 0;                 \n           } \n   }\n   \n   else if(Arr[i]==1)\n   {\n            ones = ones +1;\n            if(gnd_2==1)\n            {\n                    tick_2 = tick_2+1;\n                    gnd_2 = 0;\n                    ceil_2 = 1;\n            }\n            else \n           {\n                    tick_2 = tick_2;\n                    gnd_2 = gnd_2;\n                    ceil_2 = 1;                 \n           } \n   }\n   else\n   {\n           tick_2 = tick_2;\n           ceil_2 = ceil_2;\n           gnd_2 = gnd_2;\n   }\n}"("Arr"=w252, "size"=w258) -> ("tick_2"=w247:i32, "ones"=w246:i32)
              n180 = formula code="int i;\nint ceil_2 = 0;\nint tick_2 = 0;\nint gnd_2=0;\nint ones = 0;\n\nfor (i=0;i<size;i++)\n{\n   if(Arr[i]==0)\n   { \n            if(ceil_2==1)\n            {\n                    tick_2 = tick_2+1;\n                    gnd_2 = 1;\n                    ceil_2 = 0;\n            }\n            else \n           {\n                    tick_2 = tick_2;\n                    gnd_2 = 1;\n                    ceil_2 = 0;                 \n           } \n   }\n   \n   else if(Arr[i]==1)\n   {\n            ones = ones +1;\n            if(gnd_2==1)\n            {\n                    tick_2 = tick_2+1;\n                    gnd_2 = 0;\n                    ceil_2 = 1;\n            }\n            else \n           {\n                    tick_2 = tick_2;\n                    gnd_2 = gnd_2;\n                    ceil_2 = 1;                 \n           } \n   }\n   else\n   {\n           tick_2 = tick_2;\n           ceil_2 = ceil_2;\n           gnd_2 = gnd_2;\n   }\n}"("Arr"=w254, "size"=w256) -> ("tick_2"=w245:i32, "ones"=w244:i32)
              n181 = formula code="int i;\nint ceil_2 = 0;\nint tick_2 = 0;\nint gnd_2=0;\nint ones = 0;\n\nfor (i=0;i<size;i++)\n{\n   if(Arr[i]==0)\n   { \n            if(ceil_2==1)\n            {\n                    tick_2 = tick_2+1;\n                    gnd_2 = 1;\n                    ceil_2 = 0;\n            }\n            else \n           {\n                    tick_2 = tick_2;\n                    gnd_2 = 1;\n                    ceil_2 = 0;                 \n           } \n   }\n   \n   else if(Arr[i]==1)\n   {\n            ones = ones +1;\n            if(gnd_2==1)\n            {\n                    tick_2 = tick_2+1;\n                    gnd_2 = 0;\n                    ceil_2 = 1;\n            }\n            else \n           {\n                    tick_2 = tick_2;\n                    gnd_2 = gnd_2;\n                    ceil_2 = 1;                 \n           } \n   }\n   else\n   {\n           tick_2 = tick_2;\n           ceil_2 = ceil_2;\n           gnd_2 = gnd_2;\n   }\n}"("Arr"=w255, "size"=w259) -> ("tick_2"=w251:i32, "ones"=w250:i32)
              n182 = formula code="int i;\nint ceil_2 = 0;\nint tick_2 = 0;\nint gnd_2=0;\nint ones = 0;\n\nfor (i=0;i<size;i++)\n{\n   if(Arr[i]==0)\n   { \n            if(ceil_2==1)\n            {\n                    tick_2 = tick_2+1;\n                    gnd_2 = 1;\n                    ceil_2 = 0;\n            }\n            else \n           {\n                    tick_2 = tick_2;\n                    gnd_2 = 1;\n                    ceil_2 = 0;                 \n           } \n   }\n   \n   else if(Arr[i]==1)\n   {\n            ones = ones +1;\n            if(gnd_2==1)\n            {\n                    tick_2 = tick_2+1;\n                    gnd_2 = 0;\n                    ceil_2 = 1;\n            }\n            else \n           {\n                    tick_2 = tick_2;\n                    gnd_2 = gnd_2;\n                    ceil_2 = 1;                 \n           } \n   }\n   else\n   {\n           tick_2 = tick_2;\n           ceil_2 = ceil_2;\n           gnd_2 = gnd_2;\n   }\n}"("Arr"=w253, "size"=w257) -> ("tick_2"=w249:i32, "ones"=w248:i32)
              n183 = local read "Case_O"() -> ()  [unwired: 1 in]
              n184 = local write "var_3"(w247) -> ()
              n185 = local write "var_4"(w245) -> ()
              n186 = local write "var_1"(w251) -> ()
              n187 = local write "var_2"(w249) -> ()
              n188 = local write "Cs3_1s"(w246) -> ()
              n189 = local write "Cs4_1s"(w244) -> ()
              n190 = local write "Cs1_1s"(w250) -> ()
              n191 = local write "Cs2_1s"(w248) -> ()
            }
          }
        }
        frame Enabled {
          n192 = disable-structure shown="Enabled" {
            frame Enabled {
              n193 = flat-sequence {
                frame #0 {
                  n194 = local read "nc"() -> (w260:i32)
                  n195 = Initialize Array(0.0 ("element"), w260) -> (w262:dbl[])
                  n196 = local write "OP_Var"(w262) -> ()
                  n197 = local write "HIGH"(w262) -> ()
                }
                frame #1 {
                  n198 = local read "Case_O"() -> (w267:i32[][])
                  n199 = local read "HIGH"() -> (w266:i32[])
                  n200 = local read "OP_Var"() -> (w264:i32[])
                  n201 = local read "SD"() -> (w268:i32)
                  n202 = local read "nc"() -> (w269:i32)
                  n203 = formula code="int i, j = 0;\nint Prev_O_St = 0;\nint Curr_O_St = 0;\n\nfor (i=0;i<nc;i++)\n{\n    for(j=0; j<SD; j++)\n     {\n           if(Case_O[i][j] == 0)\n           {\n                 if(Prev_O_St == 1)\n                 {\n                       O_Var[i] = O_Var[i]  + 1;\n                       Curr_O_St = 0;\n                       Prev_O_St = Curr_O_St ;\n                 }\n                 else\n                 {\n                       O_Var[i] = O_Var[i] ;\n                       Curr_O_St = 0;\n                       Prev_O_St = Curr_O_St ;\n                 }\n           }\n            else if(Case_O[i][j] == 1)\n            {\n                  HIGH_O[i] = HIGH_O[i] + 1;\n                  if(Prev_O_St == 0)\n                 {\n                       O_Var[i] = O_Var[i]  + 1;\n                       Curr_O_St = 1;\n                       Prev_O_St = Curr_O_St ;\n                 }\n                 else\n                 {\n                       O_Var[i] = O_Var[i] ;\n                       Curr_O_St =1;\n                       Prev_O_St = Curr_O_St ;\n                 }\n             }\n\n     }\n}"("nc"=w269, "SD"=w268, "Case_O"=w267, "HIGH_O"=w266, "O_Var"=w264) -> ("HIGH_O"=w265:i32[], "O_Var"=w263:i32[])
                  "output variable" <- w265
                  n204 = local write "OP_Var"(w263) -> ()
                  n205 = local write "HIGH"(w265) -> ()
                }
              }
            }
            frame Disabled {
            }
          }
        }
      }
    }
    frame #7 {
      # "Boolean Expression Constructor"
      n206 = disable-structure shown="Enabled" {
        disable-tunnel: [w279 w463] -> w276
        frame Disabled {
          n207 = local read "N"() -> (w278:i32)
          n208 = case shown="2, Default" w278 {
            tunnel: [w300 w410] -> w280
            tunnel: [w281 w414] -> w279
            frame 2, Default {
              # "Change it from\nXOR to OR"
              n209 = local read "Cs1_1s"() -> (w317:i32)
              n210 = local read "Cs2_1s"() -> (w316:i32)
              n211 = local read "Cs3_1s"() -> (w315:i32)
              n212 = local read "Cs4_1s"() -> (w314:i32)
              n213 = case shown="1.." w315 {
                selector: w315 -> [_ w354]
                tunnel: [_ w352] -> w291
                tunnel: [_ w359] -> w303
                tunnel: [w340 w343] -> w285
                frame 0, Default {
                  n214 = local read "case3"() -> (w342:i32)
                  n215 = local read "var_3"() -> (w341:i8)
                  n216 = Divide(x=w341, y=w342) -> (x/y=w340:dbl)
                }
                frame 1.. {
                  n217 = local read "Ex_Mod_IDs"() -> (w346:string[])
                  n218 = local read "case3"() -> (w355:i32)
                  n219 = local read "var_3"() -> (w360:i8)
                  n220 = Divide(x=w360, y=w355) -> (x/y=w343:dbl)
                  n221 = Divide(x=w355, y=i8 2) -> (x/y=w358:dbl)
                  n222 = Index Array(array=w346, index=0) -> (element=w349:string)
                  n223 = Index Array(array=w346, index=1) -> (element=w347:string)
                  n224 = Less?(x=w358, y=w354) -> (x < y?=w356:bool)
                  n225 = Less?(x=w343, y=0.5) -> (x < y?=w353:bool)
                  n226 = And(x=w353, y=w356) -> (x .and. y?=w352:bool)
                  n227 = Concatenate Strings(w349, "." ("string"), w347, "!" ("string")) -> (w344:string)
                  n228 = Select(t=w344, s=w352, f="") -> (s? t:f=w359:string)
                }
              }
              n229 = case shown="1.." w317 {
                selector: w317 -> [_ w401]
                tunnel: [_ w399] -> w288
                tunnel: [_ w406] -> w307
                tunnel: [w386 w389] -> w287
                frame 0, Default {
                  n230 = local read "case1"() -> (w388:i32)
                  n231 = local read "var_1"() -> (w387:i8)
                  n232 = Divide(x=w387, y=w388) -> (x/y=w386:dbl)
                }
                frame 1.. {
                  n233 = local read "case1"() -> (w402:i32)
                  n234 = local read "var_1"() -> (w407:i8)
                  n235 = local read "Ex_Mod_IDs"() -> (w390:string[])
                  n236 = Divide(x=w407, y=w402) -> (x/y=w389:dbl)
                  n237 = Divide(x=w402, y=i8 2) -> (x/y=w405:dbl)
                  n238 = Less?(x=w389, y=0.5) -> (x < y?=w400:bool)
                  n239 = Index Array(array=w390, index=0) -> (element=w396:string)
                  n240 = Index Array(array=w390, index=1) -> (element=w393:string)
                  n241 = Less?(x=w405, y=w401) -> (x < y?=w403:bool)
                  n242 = And(x=w400, y=w403) -> (x .and. y?=w399:bool)
                  n243 = Concatenate Strings(w396, "!" ("t"), "." ("string"), w393, "!" ("t")) -> (w391:string)
                  n244 = Select(t=w391, s=w399, f="") -> (s? t:f=w406:string)
                }
              }
              n245 = case shown="1.." w316 {
                selector: w316 -> [_ w376]
                tunnel: [_ w374] -> w295
                tunnel: [_ w382] -> w305
                tunnel: [w363 w381] -> w286
                frame 0, Default {
                  n246 = local read "case2"() -> (w364:i32)
                  n247 = local read "var_2"() -> (w365:i8)
                  n248 = Divide(x=w365, y=w364) -> (x/y=w363:dbl)
                }
                frame 1.. {
                  n249 = local read "case2"() -> (w377:i32)
                  n250 = local read "var_2"() -> (w383:i8)
                  n251 = local read "Ex_Mod_IDs"() -> (w373:string[])
                  n252 = Divide(x=w383, y=w377) -> (x/y=w381:dbl)
                  n253 = Divide(x=w377, y=i8 2) -> (x/y=w378:dbl)
                  n254 = Less?(x=w381, y=0.5) -> (x < y?=w375:bool)
                  n255 = Less?(x=w378, y=w376) -> (x < y?=w380:bool)
                  n256 = Index Array(array=w373, index=0) -> (element=w369:string)
                  n257 = Index Array(array=w373, index=1) -> (element=w372:string)
                  n258 = And(x=w375, y=w380) -> (x .and. y?=w374:bool)
                  n259 = Concatenate Strings(w369, "!" ("t"), "." ("string"), w372) -> (w366:string)
                  n260 = Select(t=w366, s=w374, f="") -> (s? t:f=w382:string)
                }
              }
              n261 = case shown="1.." w314 {
                selector: w314 -> [_ w332]
                tunnel: [_ w329] -> w290
                tunnel: [_ w336] -> w301
                tunnel: [w318 w321] -> w284
                frame 0, Default {
                  n262 = local read "case4"() -> (w319:i32)
                  n263 = local read "var_4"() -> (w320:i8)
                  n264 = Divide(x=w320, y=w319) -> (x/y=w318:dbl)
                }
                frame 1.. {
                  n265 = local read "case4"() -> (w331:i32)
                  n266 = local read "var_4"() -> (w337:i8)
                  n267 = local read "Ex_Mod_IDs"() -> (w328:string[])
                  n268 = Divide(x=w337, y=w331) -> (x/y=w321:dbl)
                  n269 = Divide(x=w331, y=i8 2) -> (x/y=w333:dbl)
                  n270 = Less?(x=w321, y=0.5) -> (x < y?=w330:bool)
                  n271 = Index Array(array=w328, index=0) -> (element=w325:string)
                  n272 = Index Array(array=w328, index=1) -> (element=w327:string)
                  n273 = Less?(x=w333, y=w332) -> (x < y?=w335:bool)
                  n274 = And(x=w330, y=w335) -> (x .and. y?=w329:bool)
                  n275 = Concatenate Strings(w325, "." ("string"), w327) -> (w322:string)
                  n276 = Select(t=w322, s=w329, f="") -> (s? t:f=w336:string)
                }
              }
              n277 = And(x=w288, y=w295) -> (x .and. y?=w298:bool)
              n278 = And(x=w288, y=w291) -> (x .and. y?=w297:bool)
              n279 = And(x=w288, y=w290) -> (x .and. y?=w296:bool)
              n280 = And(x=w295, y=w291) -> (x .and. y?=w293:bool)
              n281 = And(x=w295, y=w290) -> (x .and. y?=w292:bool)
              n282 = And(x=w291, y=w290) -> (x .and. y?=w289:bool)
              n283 = Compound Arithmetic op=OR(w298, w297, w296) -> (w299:bool)
              n284 = Compound Arithmetic op=OR(w293, w292) -> (w294:bool)
              n285 = Select(t="+", s=w299, f="") -> (s? t:f=w306:string)
              n286 = Select(t="+", s=w294, f="") -> (s? t:f=w304:string)
              n287 = Select(t="+", s=w289, f="") -> (s? t:f=w302:string)
              n288 = Concatenate Strings(w307, w306, w305, w304, w303, w302, w301) -> (w300:string)
              n289 = Compound Arithmetic op=ADD(w287, w286, w285, w284) -> (w282:dbl)
              n290 = Divide(x=w282, y=4.0) -> (x/y=w281:dbl)
            }
            frame 1 {
              n291 = local read "Cs1_1s"() -> (w424:i32)
              n292 = local read "Cs2_1s"() -> (w423:i32)
              n293 = case shown="1.." w423 {
                selector: w423 -> [_ w433]
                tunnel: [_ w431] -> w420
                tunnel: [_ w439] -> w421
                tunnel: [w425 w438] -> w417
                frame 0, Default {
                  n294 = local read "case2"() -> (w426:i32)
                  n295 = local read "var_2"() -> (w427:i8)
                  n296 = Divide(x=w427, y=w426) -> (x/y=w425:dbl)
                }
                frame 1.. {
                  n297 = local read "case2"() -> (w434:i32)
                  n298 = local read "var_2"() -> (w440:i8)
                  n299 = local read "Ex_Mod_IDs"() -> (w430:string[])
                  n300 = Divide(x=w440, y=w434) -> (x/y=w438:dbl)
                  n301 = Divide(x=w434, y=i8 2) -> (x/y=w435:dbl)
                  n302 = Less?(x=w438, y=0.5) -> (x < y?=w432:bool)
                  n303 = Less?(x=w435, y=w433) -> (x < y?=w437:bool)
                  n304 = Index Array(array=w430, index=0) -> (element=w428:string)
                  n305 = And(x=w432, y=w437) -> (x .and. y?=w431:bool)
                  n306 = Select(t=w428, s=w431, f="") -> (s? t:f=w439:string)
                }
              }
              n307 = case shown="1.." w424 {
                selector: w424 -> [_ w454]
                tunnel: [_ w452] -> w419
                tunnel: [_ w459] -> w422
                tunnel: [w443 w446] -> w418
                frame 0, Default {
                  n308 = local read "case1"() -> (w445:i32)
                  n309 = local read "var_1"() -> (w444:i8)
                  n310 = Divide(x=w444, y=w445) -> (x/y=w443:dbl)
                }
                frame 1.. {
                  n311 = local read "case1"() -> (w455:i32)
                  n312 = local read "var_1"() -> (w460:i8)
                  n313 = local read "Ex_Mod_IDs"() -> (w447:string[])
                  n314 = Divide(x=w460, y=w455) -> (x/y=w446:dbl)
                  n315 = Divide(x=w455, y=i8 2) -> (x/y=w458:dbl)
                  n316 = Less?(x=w446, y=0.5) -> (x < y?=w453:bool)
                  n317 = Index Array(array=w447, index=0) -> (element=w450:string)
                  n318 = Less?(x=w458, y=w454) -> (x < y?=w456:bool)
                  n319 = And(x=w453, y=w456) -> (x .and. y?=w452:bool)
                  n320 = Concatenate Strings(w450, "!" ("t")) -> (w448:string)
                  n321 = Select(t=w448, s=w452, f="") -> (s? t:f=w459:string)
                }
              }
              n322 = Not Exclusive Or(1:w420, 2:w419) -> (0:w413:bool)
              n323 = Concatenate Strings(w422, w421) -> (w412:string)
              n324 = Select(t="", s=w413, f=w412) -> (s? t:f=w410:string)
              n325 = Compound Arithmetic op=ADD(w418, w417) -> (w415:dbl)
              n326 = Divide(x=w415, y=2.0) -> (x/y=w414:dbl)
            }
          }
          n327 = local write "Boolean  Expression"(w280) -> ()
        }
        frame Enabled {
          n328 = disable-structure shown="Enabled" {
            disable-tunnel: [w469 _] -> w463
            frame Enabled {
              # "Removing any \"+\" present at the end of BE"
              n329 = local read "N"() -> (w473:i32)
              n330 = local read "OP_Var"() -> (w482:i32[])
              n331 = local read "Case_I"() -> (w481:i32[])
              n332 = local read "HIGH"() -> (w483:i32[])
              n333 = local read "nc"() -> (w484:i32)
              n334 = Initialize Array(FALSE, w473) -> (→"Dig_In":bool[])
              n335 = Scale By Power Of 2(n=w473, x=1.0) -> (x*2^n=w476:dbl)
              n336 = for {
                N: w484 -> [_]
                tunnel: w483 -> [w617] mode=indexing
                tunnel: w482 -> [w616] mode=indexing
                tunnel: w481 -> [w615] mode=indexing
                shift-right: [w613] -> w470
                shift-left: 0.0 -> [w614]
                tunnel: [w612] -> w477 mode=indexing
                shift-right: [w605] -> w466
                shift-left: "" -> [w611]
                tunnel: [w599] -> w467 mode=indexing
                i -> [w608]
                # "0\n1\n1\n1"
                # "last\n0\n1\n0\n1"
                # "empty\n0\n0\n1\n1"
                # "down"
                # "up"
                n337 = case shown="1.." w617 {
                  selector: w617 -> [_ w753]
                  tunnel: [_ w749] -> _
                  tunnel: [w619 w748] -> w603
                  tunnel: [w624 w745] -> _
                  tunnel: w616 -> [_ w751]
                  tunnel: w615 -> [_ w750]
                  tunnel: w614 -> [_ w747]
                  tunnel: [w618 w746] -> w613
                  tunnel: w608 -> [_ w744]
                  tunnel: [w623 w743] -> w612
                  tunnel: w611 -> [w620 w742]
                  tunnel: [FALSE ("x .and. y?") w741] -> w599
                  frame 0, Default {
                    n338 = local read "Dig_In"() -> (w623:bool[])
                    n339 = xnode "Match Regular Expression"("input string"=w620, "regular expression"="\\+$") -> ("before match"=w619:string)  [unwired: 4 in, 4 out]
                    n340 = local read "case1"() -> (w626:i32)
                    n341 = local read "var_1"() -> (w625:i8)
                    n342 = local read "TV"() -> (w618:dbl)
                    n343 = Divide(x=w625, y=w626) -> (x/y=w624:dbl)
                  }
                  frame 1.. {
                    n344 = Divide(x=w751, y=w750) -> (x/y=w745:dbl)
                    n345 = Divide(x=w750, y=i8 2) -> (x/y=w756:dbl)
                    n346 = Less?(x=w745, y=0.5) -> (x < y?=w752:bool)
                    n347 = Less?(x=w756, y=w753) -> (x < y?=w754:bool)
                    n348 = And(x=w752, y=w754) -> (x .and. y?=w749:bool)
                    n349 = case shown="False" w749 {
                      tunnel: [w758 w879] -> w748
                      tunnel: w744 -> [_ w883]
                      tunnel: [w762 w881] -> w743
                      tunnel: w742 -> [w759 w878]
                      tunnel: [FALSE ("x .and. y?") TRUE ("x .and. y?")] -> w741
                      frame False {
                        n350 = local read "Dig_In"() -> (w762:bool[])
                        n351 = xnode "Match Regular Expression"("input string"=w759, "regular expression"="\\+$") -> ("before match"=w758:string)  [unwired: 4 in, 4 out]
                      }
                      frame True {
                        n352 = Number To Boolean Array(number=w883) -> (Boolean array=w884:bool[])
                        n353 = local read "N"() -> (w882:i32)
                        n354 = Reverse 1D Array(array=w884) -> (reversed array=w885:bool[])
                        n355 = Array Size(array=w885) -> (size(s)=w886:i32)
                        n356 = Subtract(x=w886, y=w882) -> (x-y=w887:i32)
                        n357 = Array Subset(array=w885, index=w887, length=w882) -> (w881:bool[])
                        n358 = local read "Ex_Mod_IDs"() -> (w880:string[])
                        n359 = for {
                          N -> [w897]
                          tunnel: w881 -> [w901] mode=indexing
                          tunnel: w880 -> [w900] mode=indexing
                          shift-right: [w891] -> w879
                          shift-left: w878 -> [w890]
                          i -> [w896]
                          n360 = Concatenate Strings(w900, "'" ("string")) -> (w898:string)
                          n361 = Decrement(x=w897) -> (x-1=w895:i32)
                          n362 = Select(t=w900, s=w901, f=w898) -> (s? t:f=w889:string)
                          n363 = Equal?(x=w895, y=w896) -> (x = y?=w894:bool)
                          n364 = Concatenate Strings(w890, w889) -> (w888:string)
                          n365 = Concatenate Strings(w888, ".") -> (w893:string)
                          n366 = Select(t=w888, s=w894, f=w893) -> (s? t:f=w891:string)
                        }
                        n367 = local write "Int_BE"(w879) -> ()
                      }
                    }
                    n368 = Add(x=w745, y=w747) -> (x+y=w746:dbl)
                    n369 = local write "TV"(w746) -> ()
                  }
                }
                n370 = local read "nc"() -> (w609:i32)
                n371 = Decrement(x=w609) -> (x-1=w610:i32)
                n372 = Equal?(x=w610, y=w608) -> (x = y?=w601:bool)
                n373 = Equal?(x=w603, y="") -> (x = y?=w602:bool)
                n374 = Or(x=w601, y=w602) -> (x .or. y?=w600:bool)
                n375 = Concatenate Strings(w603, "+") -> (w606:string)
                n376 = Select(t=w603, s=w600, f=w606) -> (s? t:f=w605:string)
              }
              "Array 2" <- w477
              "Output Array" <- w467
              n377 = Initialize Array(FALSE, w476, w473) -> (w472:bool[][])
              n378 = local write "Array 2"(w472) -> ()
              n379 = Divide(x=w470, y=4.0) -> (x/y=w469:dbl)
              n380 = xnode "Match Regular Expression"("input string"=w466, "regular expression"="\\+$") -> ("before match"=w464:string)  [unwired: 4 in, 4 out]
              n381 = local write "Final_BE"(w464) -> ()
              n382 = local write "Boolean  Expression"(w464) -> ()
            }
            frame Disabled {
            }
          }
        }
      }
      n383 = Multiply(x=w276, y=100.0) -> (x*y=w274:dbl)
      n384 = Subtract(x=100.0 ("y"), y=w274) -> (x-y=w272:dbl)
      n385 = Number To Fractional String(number=w272, precision (6)=i16 2) -> (F-format string=w273:string)  [unwired: 2 in]
      n386 = case shown="Default" w273 {
        selector: w273 -> [w904 _]
        tunnel: [w903 "All input combinations are not applied correctly!" ("% fitness")] -> w271
        frame Default {
          n387 = local read "Input Status"() -> (w902:bool)
          n388 = case shown="False" w902 {
            tunnel: w904 -> [w909 _]
            tunnel: [w908 "All input combinations are not applied correctly!" ("% fitness")] -> w903
            frame False {
              n389 = local read "Final_BE"() -> (w906:string)
              n390 = Not Equal?(x=w906, y="") -> (x != y?=w905:bool)
              n391 = case shown="True" w905 {
                tunnel: w909 -> [_ w917]
                tunnel: ["Error" ("% fitness") w916] -> w908
                frame False {
                  n392 = property on="% fitness" class="Str"("Text.TextColor"=u32 15670016) -> ()  [unwired: 2 in, 2 out]
                  n393 = property on="% fitness" class="Str"("Text.FontSize"=u32 18 ("Text.Font:Size")) -> ()  [unwired: 2 in, 2 out]
                }
                frame True {
                  n394 = property on="% fitness" class="Str"("Text.FontSize"=u32 20 ("Text.Font:Size")) -> ()  [unwired: 2 in, 2 out]
                  n395 = property on="% fitness" class="Str"("Text.TextColor"=u32 2846208) -> ()  [unwired: 2 in, 2 out]
                  n396 = Concatenate Strings("Fitness = ", w917, " %" ("string")) -> (w916:string)
                }
              }
            }
            frame True {
              n397 = property on="% fitness" class="Str"("Text.TextColor"=u32 15670016) -> ()  [unwired: 2 in, 2 out]
              n398 = property on="% fitness" class="Str"("Text.FontSize"=u32 18 ("Text.Font:Size")) -> ()  [unwired: 2 in, 2 out]
            }
          }
        }
        frame "NaN" {
          n399 = property on="% fitness" class="Str"("Text.TextColor"=u32 15670016) -> ()  [unwired: 2 in, 2 out]
          n400 = property on="% fitness" class="Str"("Text.FontSize"=u32 18 ("Text.Font:Size")) -> ()  [unwired: 2 in, 2 out]
        }
      }
      n401 = local write "% fitness"(w271) -> ()
    }
    frame #8 {
      # "Remove Empty strings and replace it with the previous expressions"
      n402 = disable-structure shown="Disabled" {
        frame Disabled {
          n403 = local read "Boolean  Expression"() -> (w930:string)
          n404 = local read "Ex_Mod_IDs"() -> (w941:string[])
          n405 = call "2-input AND.vi"("Obtained Expression"=w930, "Input List"=w941) -> ("AND ?"=w946:bool, "Logic Exp"=w947:string)  [unwired: 7 in, 1 out]
          n406 = call "2-input NAND.vi"("Obtained Expression"=w930, "Input List"=w941) -> ("NAND ?"=w956:bool, "Logic Exp"=w951:string)  [unwired: 7 in, 1 out]
          n407 = call "2-input OR.vi"("Obtained Expression"=w930, "Input List"=w941) -> ("OR ?"=w955:bool, "Logic Exp"=w952:string)  [unwired: 7 in, 1 out]
          n408 = call "2-input NOR.vi"("Obtained Expression"=w930, "Input List"=w941) -> ("Nand ?"=w954:bool, "Logic Exp"=w953:string)  [unwired: 7 in, 1 out]
          n409 = call "2-input NOT.vi"("Obtained Expression"=w930, "Input List"=w941) -> ("NOT ?"=w942:bool, "Logic Exp"=w943:string)  [unwired: 7 in, 1 out]
          n410 = Select(t=w947, s=w946, f="") -> (s? t:f=w945:string)
          n411 = Select(t=w951, s=w956, f="") -> (s? t:f=w948:string)
          n412 = Select(t=w952, s=w955, f="") -> (s? t:f=w949:string)
          n413 = Select(t=w953, s=w954, f="") -> (s? t:f=w950:string)
          n414 = Select(t=w943, s=w942, f="") -> (s? t:f=w940:string)
          n415 = local read "Boolean  Expression"() -> (w932:string)
          n416 = Concatenate Strings(w945, w948, w949, w950, w940) -> (w931:string)
          n417 = Equal?(x=w931, y="") -> (x = y?=w934:bool)
          n418 = Select(t=w932, s=w934, f=w931) -> (s? t:f=w933:string)
          n419 = local write "Boolean  Expression"(w933) -> ()
        }
        frame Enabled {
        }
      }
      n420 = local read "Output Array"() -> (w926:bool[])
      n421 = Array Size(array=w926) -> (size(s)=w927:i32)
      n422 = Decrement(x=w927) -> (x-1=w929:i32)
      n423 = Index Array(array=w926, index=w929) -> (element=w928:bool)
      "element" <- w928
      n424 = case shown="False" w928 {
        tunnel: w927 -> [w958 w1022]
        tunnel: w926 -> [w959 w1019]
        tunnel: [w957 w1018] -> w925
        frame False {
          # "It could be NAND or NOR logic"
          n425 = Subtract(x=w958, y=2) -> (x-y=w960:i32)
          n426 = Index Array(array=w959, index=w960) -> (element=w961:bool)
          n427 = case shown="False" w961 {
            tunnel: w959 -> [w963 w990]
            tunnel: [w965 w992] -> w957
            tunnel: w960 -> [w964 w991]
            frame True {
              # "This can not be NOR logic. It may be NAND"
              n428 = Index Array(array=w963, index=0) -> (element=w966:bool)
              n429 = case shown="True" w966 {
                tunnel: [w968 w969] -> w965
                tunnel: w964 -> [_ w974]
                tunnel: w963 -> [_ w972]
                frame False {
                  # "This is not NAND Gate. Output the entire BE as is."
                  n430 = local read "Boolean  Expression"() -> (w968:string)
                }
                frame True {
                  # "This may be NAND gate. Check rest of all other combinations if they are true. If not, then reflect the entire BE as is."
                  n431 = Array Subset(array=w972, index=1, length=w974) -> (w971:bool[])
                  n432 = And Array Elements(Boolean array=w971) -> (logical AND=w970:bool)
                  n433 = case shown="True" w970 {
                    tunnel: [w975 w976] -> w969
                    frame False {
                      # "This is not NAND Gate. Output BE as is"
                      n434 = local read "Boolean  Expression"() -> (w975:string)
                    }
                    frame True {
                      # "This is NAND gate"
                      n435 = local read "Ex_Mod_IDs"() -> (w982:string[])
                      n436 = for {
                        tunnel: w982 -> [w985] mode=indexing
                        shift-right: [w983] -> w980
                        shift-left: "" -> [w988]
                        i -> [w987]
                        n437 = Concatenate Strings(w988, "." ("string"), w985) -> (w984:string)
                        n438 = Equal To 0?(x=w987) -> (x = 0?=w986:bool)
                        n439 = Select(t=w985, s=w986, f=w984) -> (s? t:f=w983:string)
                      }
                      n440 = Concatenate Strings("(" ("string"), w980, ")" ("string"), "'" ("string")) -> (w976:string)
                    }
                  }
                }
              }
            }
            frame False {
              # "This can not be NAND logic. It may be NOR"
              n441 = Index Array(array=w990, index=0) -> (element=w993:bool)
              n442 = case shown="True" w993 {
                tunnel: [w995 w996] -> w992
                tunnel: w991 -> [_ w1001]
                tunnel: w990 -> [_ w999]
                frame False {
                  # "This is not NOR Gate. Output the entire BE as is."
                  n443 = local read "Boolean  Expression"() -> (w995:string)
                }
                frame True {
                  # "This may be NOR gate. Check rest of all other combinations if they are false. If not, then reflect the entire BE as is."
                  n444 = Array Subset(array=w999, index=1, length=w1001) -> (w998:bool[])
                  n445 = Or Array Elements(Boolean array=w998) -> (logical OR=w997:bool)
                  n446 = case shown="False" w997 {
                    tunnel: [w1002 w1016] -> w996
                    frame False {
                      # "This is NOR gate"
                      n447 = local read "Ex_Mod_IDs"() -> (w1008:string[])
                      n448 = for {
                        tunnel: w1008 -> [w1011] mode=indexing
                        shift-right: [w1009] -> w1003
                        shift-left: "" -> [w1014]
                        i -> [w1013]
                        n449 = Concatenate Strings(w1014, "+" ("string"), w1011) -> (w1010:string)
                        n450 = Equal To 0?(x=w1013) -> (x = 0?=w1012:bool)
                        n451 = Select(t=w1011, s=w1012, f=w1010) -> (s? t:f=w1009:string)
                      }
                      n452 = Concatenate Strings("(" ("string"), w1003, ")" ("string"), "'" ("string")) -> (w1002:string)
                    }
                    frame True {
                      # "This is not NOR gate. Output BE as is"
                      n453 = local read "Boolean  Expression"() -> (w1016:string)
                    }
                  }
                }
              }
            }
          }
        }
        frame True {
          # "It could be AND or OR logic"
          n454 = Subtract(x=w1022, y=2) -> (x-y=w1017:i32)
          n455 = Index Array(array=w1019, index=w1017) -> (element=w1020:bool)
          n456 = case shown="False" w1020 {
            tunnel: w1019 -> [w1023 w1046]
            tunnel: [w1025 w1048] -> w1018
            tunnel: w1017 -> [w1024 w1047]
            frame True {
              # "This can not be AND logic. It may be OR"
              n457 = Index Array(array=w1023, index=0) -> (element=w1026:bool)
              n458 = case shown="False" w1026 {
                tunnel: [w1028 w1045] -> w1025
                tunnel: w1024 -> [w1033 _]
                tunnel: w1023 -> [w1031 _]
                frame False {
                  # "This may be OR gate. Check rest of all other combinations if they are true. If not, then reflect the entire BE as is."
                  n459 = Array Subset(array=w1031, index=1, length=w1033) -> (w1030:bool[])
                  n460 = And Array Elements(Boolean array=w1030) -> (logical AND=w1029:bool)
                  n461 = case shown="True" w1029 {
                    tunnel: [w1034 w1035] -> w1028
                    frame False {
                      # "This is not OR Gate. Output BE as is"
                      n462 = local read "Boolean  Expression"() -> (w1034:string)
                    }
                    frame True {
                      # "This is OR gate"
                      n463 = local read "Ex_Mod_IDs"() -> (w1037:string[])
                      n464 = for {
                        tunnel: w1037 -> [w1040] mode=indexing
                        shift-right: [w1038] -> w1035
                        shift-left: "" -> [w1043]
                        i -> [w1042]
                        n465 = Concatenate Strings(w1043, "+" ("string"), w1040) -> (w1039:string)
                        n466 = Equal To 0?(x=w1042) -> (x = 0?=w1041:bool)
                        n467 = Select(t=w1040, s=w1041, f=w1039) -> (s? t:f=w1038:string)
                      }
                    }
                  }
                }
                frame True {
                  # "This is not OR Gate. Output the entire BE as is."
                  n468 = local read "Boolean  Expression"() -> (w1045:string)
                }
              }
            }
            frame False {
              # "This can not be OR logic. It may be AND"
              n469 = Index Array(array=w1046, index=0) -> (element=w1049:bool)
              n470 = case shown="False" w1049 {
                tunnel: [w1051 w1068] -> w1048
                tunnel: w1047 -> [w1056 _]
                tunnel: w1046 -> [w1054 _]
                frame False {
                  # "This may be AND gate. Check rest of all other combinations if they are false. If not, then reflect the entire BE as is."
                  n471 = Array Subset(array=w1054, index=1, length=w1056) -> (w1053:bool[])
                  n472 = Or Array Elements(Boolean array=w1053) -> (logical OR=w1052:bool)
                  n473 = case shown="False" w1052 {
                    tunnel: [w1057 w1067] -> w1051
                    frame False {
                      # "This is AND gate"
                      n474 = local read "Ex_Mod_IDs"() -> (w1059:string[])
                      n475 = for {
                        tunnel: w1059 -> [w1062] mode=indexing
                        shift-right: [w1060] -> w1057
                        shift-left: "" -> [w1065]
                        i -> [w1064]
                        n476 = Concatenate Strings(w1065, "." ("string"), w1062) -> (w1061:string)
                        n477 = Equal To 0?(x=w1064) -> (x = 0?=w1063:bool)
                        n478 = Select(t=w1062, s=w1063, f=w1061) -> (s? t:f=w1060:string)
                      }
                    }
                    frame True {
                      # "This is not AND Gate. Output BE as is"
                      n479 = local read "Boolean  Expression"() -> (w1067:string)
                    }
                  }
                }
                frame True {
                  # "This is not AND Gate. Output the entire BE as is."
                  n480 = local read "Boolean  Expression"() -> (w1068:string)
                }
              }
            }
          }
        }
      }
      n481 = local write "Boolean  Expression"(w925) -> ()
    }
    frame #9 {
      n482 = Get Date/Time In Seconds() -> (seconds since 1Jan1904=w1071:timestamp)
      n483 = Subtract(x=w1071, y=w1069) -> (x-y=w1070:dbl)
      "Estimation Time (s)" <- w1070
      n484 = disable-structure shown="Enabled" {
        disable-tunnel: w1070 -> [_ _]
        frame Enabled {
          n485 = while {
            tunnel: ["Close"] -> w1073
            stop <- "Close" stop-if-true
            n486 = Wait Until Next ms Multiple(millisecond multiple=u32 1) -> ()  [unwired: 1 out]
          }
          "Close 2" <- w1073
          n487 = Not(x=w1073) -> (.not. x?=w1072:bool)
          n488 = property class="VI"("Front Panel Window:Open"=w1072) -> ()  [unwired: 2 in, 2 out]
        }
        frame Disabled {
        }
      }
    }
  }
